vi "Steuerprogramm10-14.vi"() -> ()   [LabVIEW 2010]
uses:
  <vilib>/rvi/interface/nirviReadWriteControl/nirviReadWriteControl.xnode
  <vilib>/rvi/errors/niLvFpgaWhatHappensToTopLevelVI.ctl
  <vilib>/rvi/interface/common/niFpgaNodeNameForErrorReporting.ctl
  <vilib>/rvi/errors/niLvFpgaAdjustHostInterfaceError.vi
  gvbooleschRT.vi
  <vilib>/functionblocks/FB Core/FB Core.xnode
  <vilib>/functionblocks/Counter/Elapsed Timer/Elapsed Timer.vi
  <vilib>/functionblocks/NI_FunctionBlock Libraries.lvlib
  <vilib>/rvi/interface/nirviCloseFPGA/nirviCloseFPGA.xnode
  <vilib>/addons/control/pid/NI_PID_pid.lvlib
  C:/Users/HAGAR-IV/Desktop/Zeugs/Johnny/pertrasgc fpga/FPGA-Programm-10-14.vi
  C:/Users/HAGAR-IV/Desktop/Zeugs/markus/version feb 2012/FPGA Bitfiles/pertrasgcfpga2_FPGATarget_FPGA-Programm-10_16368CB6.lvbitx
  <vilib>/addons/control/pid/pid.llb/PID (DBL Array).vi
  NiFpgaLv.dll
  <vilib>/Utility/error.llb/Error Cluster From Error Code.vi
  <vilib>/FPGAPlugInAG/cRIO-9114/niLvFpga_Close_cRIO-9114.vi
panel:
  in  "Int.Stop2":dbl
  in  "Int.Start2":dbl
  out "Probenvol.2":dbl
  in  "Int.Stop1":dbl
  in  "Int.Start1":dbl
  in  "HorstProbenflußNr.":i32
  out "AIs":dbl[](array[numeric])
  out "Probenvol.1":dbl
  in  "Eingang":T1(array[cluster])=[{"Zykluslängen [s]"=[120.0, 120.0, 120.0, 120.0], "ZeitpktDIOsMod0"=[0.0, 120.0], "ZeitpktDIOsMod1"=[0.0, 60.0, 62.0, 70.0, 120.0], "ZeitpktDIOsMod2A"=[0.0, 120.0], "ZeitpktDIOsMod2B"=[0.0, 60.0, 120.0], "DIOsSPMod0"=[[FALSE], [FALSE]], "DIOsSPMod1"=[[FALSE, FALSE, FALSE, FALSE, FALSE, TRUE, TRUE, FALSE, FALSE, FALSE, TRUE, FALSE, FALSE, FALSE, FALSE, FALSE, FALSE, FALSE], [FALSE, FALSE, FALSE, FALSE, FALSE, FALSE, TRUE, FALSE, FALSE, FALSE, FALSE, FALSE, FALSE, FALSE, FALSE, FALSE, TRUE, FALSE], [FALSE, FALSE, FALSE, FALSE, FALSE, FALSE, TRUE, FALSE, FALSE, FALSE, TRUE, FALSE, FALSE, FALSE, FALSE, FALSE, TRUE, FALSE], [FALSE, FALSE, FALSE, FALSE, FALSE, FALSE, TRUE, FALSE, FALSE, FALSE, TRUE, FALSE, FALSE, FALSE, FALSE, FALSE, FALSE, FALSE], [FALSE, FALSE, FALSE, FALSE, FALSE, FALSE, TRUE, FALSE, FALSE, FALSE, TRUE, FALSE, FALSE, FALSE, FALSE, FALSE, FALSE, FALSE]], "DIOsSPMod2A"=[[FALSE], [FALSE]], "DIOsSPMod2B"=[[FALSE], [FALSE]], "Mod0HorstZeitpkt"=[0.0, 120.0], "Mod1HorstZeitpkt"=[0.0, 59.0, 62.0, 120.0], "Mod2AHorstZeitpkt"=[0.0, 120.0], "Mod2BHorstZeitpkt"=[0.0, 120.0], "HorstSPMod0"=[[0.0], [0.0]], "HorstSPMod1"=[[3.0, 0.0, 0.8], [0.0, 0.0, 0.8], [1.0, 0.0, 0.8], [1.0, 0.0, 0.8]], "HorstSPMod2A"=[[0.0], [0.0]], "HorstSPMod2B"=[[0.0], [0.0]], "LangsameHeizungenSP"=[0.0, 100.0, 100.0, 0.0, 0.0, 0.0], "LHHeizen?"=[FALSE, TRUE, FALSE, FALSE, FALSE, FALSE], "ZPktFPGABoolesch"=[0.0, 62.0, 70.0, 120.0], "FPGABoolesch"=[[FALSE, FALSE, FALSE, FALSE, FALSE, FALSE], [FALSE, FALSE, TRUE, FALSE, FALSE, FALSE], [FALSE, FALSE, FALSE, FALSE, FALSE, FALSE], [FALSE, FALSE, FALSE, FALSE, FALSE, FALSE]], "ZeitpktFPGAPID"=[0.0, 120.0], "FPGAPID"=[[{"proportional gain (Kc)"=1.0, "integral gain (Kc*Ts/Ti)"=1.66796875, "derivative gain (Kc*Td/Ts)"=0.0}, {"proportional gain (Kc)"=1.0, "integral gain (Kc*Ts/Ti)"=1.66796875, "derivative gain (Kc*Td/Ts)"=0.0}, {"proportional gain (Kc)"=5.0, "integral gain (Kc*Ts/Ti)"=0.03515625, "derivative gain (Kc*Td/Ts)"=0.0234375}, {"proportional gain (Kc)"=1.0, "integral gain (Kc*Ts/Ti)"=1.66796875, "derivative gain (Kc*Td/Ts)"=0.0}], [{"proportional gain (Kc)"=1.0, "integral gain (Kc*Ts/Ti)"=1.66796875, "derivative gain (Kc*Td/Ts)"=0.0}, {"proportional gain (Kc)"=1.0, "integral gain (Kc*Ts/Ti)"=1.66796875, "derivative gain (Kc*Td/Ts)"=0.0}, {"proportional gain (Kc)"=5.0, "integral gain (Kc*Ts/Ti)"=0.03515625, "derivative gain (Kc*Td/Ts)"=0.0234375}, {"proportional gain (Kc)"=1.0, "integral gain (Kc*Ts/Ti)"=1.66796875, "derivative gain (Kc*Td/Ts)"=0.0}], [{"proportional gain (Kc)"=0.0, "integral gain (Kc*Ts/Ti)"=0.0, "derivative gain (Kc*Td/Ts)"=0.0}, {"proportional gain (Kc)"=0.0, "integral gain (Kc*Ts/Ti)"=0.0, "derivative gain (Kc*Td/Ts)"=0.0}, {"proportional gain (Kc)"=5.0, "integral gain (Kc*Ts/Ti)"=0.03125, "derivative gain (Kc*Td/Ts)"=0.01953125}, {"proportional gain (Kc)"=0.0, "integral gain (Kc*Ts/Ti)"=0.0, "derivative gain (Kc*Td/Ts)"=0.0}], [{"proportional gain (Kc)"=0.0, "integral gain (Kc*Ts/Ti)"=0.0, "derivative gain (Kc*Td/Ts)"=0.0}, {"proportional gain (Kc)"=0.0, "integral gain (Kc*Ts/Ti)"=0.0, "derivative gain (Kc*Td/Ts)"=0.0}, {"proportional gain (Kc)"=5.0, "integral gain (Kc*Ts/Ti)"=0.03125, "derivative gain (Kc*Td/Ts)"=0.01953125}, {"proportional gain (Kc)"=0.0, "integral gain (Kc*Ts/Ti)"=0.0, "derivative gain (Kc*Td/Ts)"=0.0}], [{"proportional gain (Kc)"=0.0, "integral gain (Kc*Ts/Ti)"=0.0, "derivative gain (Kc*Td/Ts)"=0.0}, {"proportional gain (Kc)"=0.0, "integral gain (Kc*Ts/Ti)"=0.0, "derivative gain (Kc*Td/Ts)"=0.0}, {"proportional gain (Kc)"=5.0, "integral gain (Kc*Ts/Ti)"=0.03125, "derivative gain (Kc*Td/Ts)"=0.01953125}, {"proportional gain (Kc)"=0.0, "integral gain (Kc*Ts/Ti)"=0.0, "derivative gain (Kc*Td/Ts)"=0.0}]], "ZeitpktFPGAFixp"=[0.0, 120.0], "FPGAFixp"=[[3.5, 3.5, 1.800048828125, 0.0, 0.0, 0.0, 2.400146484375, 0.0], [3.5, 3.5, 1.800048828125, 0.0, 0.0, 0.0, 2.400146484375, 0.0]], "ZeitpktMach1"=[0.0, 65.0, 72.0, 110.0, 111.0, 120.0], "TempMach1"=[70.0, 70.0, 150.0, 150.0, 70.0, 70.0], "ZeitpktMach2"=[0.0, 0.0, 120.0], "TempMach2"=[0.0, 0.0, 0.0], "PIDs für \"träge\" Heizungen"=[{"proportional gain (Kc)"=1.0, "integral time (Ti, min)"=0.01, "derivative time (Td, min)"=0.0}, {"proportional gain (Kc)"=5.0, "integral time (Ti, min)"=5.0, "derivative time (Td, min)"=5.0}, {"proportional gain (Kc)"=5.0, "integral time (Ti, min)"=1.0, "derivative time (Td, min)"=5.0}, {"proportional gain (Kc)"=1.0, "integral time (Ti, min)"=0.01, "derivative time (Td, min)"=0.0}, {"proportional gain (Kc)"=1.0, "integral time (Ti, min)"=0.01, "derivative time (Td, min)"=0.0}, {"proportional gain (Kc)"=1.0, "integral time (Ti, min)"=0.01, "derivative time (Td, min)"=0.0}], "Zwangsbedingungen"=[[0.0, 0.0, 0.0, 0.0, 0.0]], "Text0 MS-Datei"="text0", "Info"="info", "wie wird gespeichert?"=0, "Speicherlänge"="100", "Dateien fürs MS schicken?"=FALSE, "Pfad MS-Datei CRIO"=path "c:/"}] {"FPGAPID"."proportional gain (Kc)" format="%.11g"; "FPGAPID"."integral gain (Kc*Ts/Ti)" format="%.11g"; "FPGAPID"."derivative gain (Kc*Td/Ts)" format="%.11g"; "FPGAFixp" format="%.14g"}
  out "Ausgang":T2 {"FPGAPID"."proportional gain (Kc)" format="%.11g"; "FPGAPID"."integral gain (Kc*Ts/Ti)" format="%.11g"; "FPGAPID"."derivative gain (Kc*Td/Ts)" format="%.11g"; "FPGAFixp" format="%.14g"}
  out "Zykluslängen [s]":dbl[](array[numeric])
  in  "Tafel putzen1":bool
  in  "Tafel putzen2":bool
  in  "veränderte Methode benutzen":bool
  out "veränderte Methode":T2 {"FPGAPID"."proportional gain (Kc)" format="%.11g"; "FPGAPID"."integral gain (Kc*Ts/Ti)" format="%.11g"; "FPGAPID"."derivative gain (Kc*Td/Ts)" format="%.11g"; "FPGAFixp" format="%.14g"}
  in  "Methode verändern":bool
  in  "dargestellte Größe 2":i32(ring)=1 items=["T-MainCol3", "T-Trap1", "T-Trap2", "T-Stirling", "T-PreCol1", "T-PreCol2", "T-MainCol1", "T-MainCol2", "T-T-Line2", "T-MI1", "T-MI2", "T-MI3", "T-MI4", "T-MI5", "T-MI6", "F-MFM1", "T-MainCol4", "T-BHorst1", "T-BHorst2", "T-BHorst3", "T-BHorst4", "T-Oven1", "T-Oven2", "T-T-Line1", "F-MFM2", "P-Me-HP", "P-Me-LP", "P-Vac", "Ref-Turbo", "I-MS-AC", "I-Trap1", "I-Trap2", "Mod2/AI0", "Mod2/AI1", "Mod2/AI2", "Mod2/AI3", "Mod2/AI4", "Mod2/AI5", "Mod2/AI6", "Mod2/AI7", "Mod2/AI8", "Mod2/AI9", "Mod2/AI10", "Mod2/AI11", "Mod2/AI12", "Mod2/AI13", "Mod2/AI14", "Mod2/AI15", "Mod2/AI16", "Mod2/AI17", "Mod2/AI18", "Mod2/AI19", "Mod2/AI20", "Mod2/AI21", "Mod2/AI22", "Mod2/AI23", "Mod2/AI24", "Mod2/AI25", "Mod2/AI26", "Mod2/AI27", "Mod2/AI28", "Mod2/AI29", "Mod2/AI30", "Mod2/AI31", "Mod3/AI0", "Mod3/AI1", "Mod3/AI2", "Mod3/AI3", "Mod3/AI4", "Mod3/AI5", "Mod3/AI6", "Mod3/AI7", "Mod3/AI8", "Mod3/AI9", "Mod3/AI10", "Mod3/AI11", "Mod3/AI12", "Mod3/AI13", "Mod3/AI14", "Mod3/AI15", "Mod3/AI16", "Mod3/AI17", "Mod3/AI18", "Mod3/AI19", "Mod3/AI20", "Mod3/AI21", "Mod3/AI22", "Mod3/AI23", "Mod3/AI24", "Mod3/AI25", "Mod3/AI26", "Mod3/AI27", "Mod3/AI28", "Mod3/AI29", "Mod3/AI30", "Mod3/AI31", "U_Widr.Trap1 [V]", "Temp.Trap1 [°C]", "U_Widr.Trap2 [V]", "Temp.Trap2 [°C]", "Temp.Mach1 [°C]", "Temp.Mach2 [°C]", "MFC1B", "PressContr1A", "PressContr1B", "PressContr1C", "MFC1A", "PressContr1D", "MFC1A Integriert"]
  in  "Zeitachse2":i32(ring)=1 items=["Zykluszeit [s] Mod0", "Zykluszeit [s] Mod1", "Zykluszeit [s] Mod2A", "Zykluszeit [s] Mod2B"]
  out "Anzeige2":cluster{dbl[], dbl[]}(graph)
  out "Datum/Zeit":string
  in  "wie wird gespeichert?":u16(ring) items=["Time", "Cycle", "All"]
  in  "Info":string
  in  "Speicherlänge":string
  in  "Dateien fürs MS schicken?":bool
  in  "Pfad MS-Datei CRIO":path
  in  "Text0 MS-Datei":string
  out "ZwangsHorst!":cluster{dbl[]}[](array[cluster])
  out "ZwangsHorst?":cluster{bool[]}[](array[cluster])
  out "ZwangsDIO!":cluster{bool[]}[](array[cluster])
  out "ZwangsDIO?":cluster{bool[]}[](array[cluster])
  out "PIDs für \"träge\" Heizungen":T3(array[cluster])
  out "ZwangsLangsameH!":bool[](array[boolean])
  in  "Heizen?LH":bool[](array[boolean])
  out "Zwangsbedingungen":dbl[][](array[numeric])
  out "Traps/Machs":dbl[](array[numeric])
  out "ZwangsFPGABoolesch!":bool[](array[boolean])
  out "ZwangsFPGABoolesch?":bool[](array[boolean])
  in  "LangsameHeizungenSP":dbl[](array[numeric])
  out "ZwangsLangsameH?":bool[](array[boolean])
  out "Zykluszeiten 0, 1, 2A, 2B":dbl[](array[numeric])
  out "Zyklusnummern 0, 1, 2A, 2B":i32[](array[numeric])
  in  "dargestellte Größe 1":i32(ring)=1 items=["T-MainCol3", "T-Trap1", "T-Trap2", "T-Stirling", "T-PreCol1", "T-PreCol2", "T-MainCol1", "T-MainCol2", "T-T-Line2", "T-MI1", "T-MI2", "T-MI3", "T-MI4", "T-MI5", "T-MI6", "F-MFM1", "T-MainCol4", "T-BHorst1", "T-BHorst2", "T-BHorst3", "T-BHorst4", "T-Oven1", "T-Oven2", "T-T-Line1", "F-MFM2", "P-Me-HP", "P-Me-LP", "P-Vac", "Ref-Turbo", "I-MS-AC", "I-Trap1", "I-Trap2", "Mod2/AI0", "Mod2/AI1", "Mod2/AI2", "Mod2/AI3", "Mod2/AI4", "Mod2/AI5", "Mod2/AI6", "Mod2/AI7", "Mod2/AI8", "Mod2/AI9", "Mod2/AI10", "Mod2/AI11", "Mod2/AI12", "Mod2/AI13", "Mod2/AI14", "Mod2/AI15", "Mod2/AI16", "Mod2/AI17", "Mod2/AI18", "Mod2/AI19", "Mod2/AI20", "Mod2/AI21", "Mod2/AI22", "Mod2/AI23", "Mod2/AI24", "Mod2/AI25", "Mod2/AI26", "Mod2/AI27", "Mod2/AI28", "Mod2/AI29", "Mod2/AI30", "Mod2/AI31", "Mod3/AI0", "Mod3/AI1", "Mod3/AI2", "Mod3/AI3", "Mod3/AI4", "Mod3/AI5", "Mod3/AI6", "Mod3/AI7", "Mod3/AI8", "Mod3/AI9", "Mod3/AI10", "Mod3/AI11", "Mod3/AI12", "Mod3/AI13", "Mod3/AI14", "Mod3/AI15", "Mod3/AI16", "Mod3/AI17", "Mod3/AI18", "Mod3/AI19", "Mod3/AI20", "Mod3/AI21", "Mod3/AI22", "Mod3/AI23", "Mod3/AI24", "Mod3/AI25", "Mod3/AI26", "Mod3/AI27", "Mod3/AI28", "Mod3/AI29", "Mod3/AI30", "Mod3/AI31", "U_Widr.Trap1 [V]", "Temp.Trap1 [°C]", "U_Widr.Trap2 [V]", "Temp.Trap2 [°C]", "Temp.Mach1 [°C]", "Temp.Mach2 [°C]", "MFC1B", "PressContr1A", "PressContr1B", "PressContr1C", "MFC1A", "PressContr1D", "MFC1A Integriert"]
  in  "Zeitachse1":i32(ring)=1 items=["Zykluszeit [s] Mod0", "Zykluszeit [s] Mod1", "Zykluszeit [s] Mod2A", "Zykluszeit [s] Mod2B"]
  out "Anzeige1":cluster{dbl[], dbl[]}(graph)
  out "Big Ben, Methodenzeit, Zykluszeit0, Zykluszeit1, Zykluszeit2A, Zykluszeit2B":dbl[](array[numeric])
  out "MWHorst":dbl[](array[numeric])
  out "HorstSP":dbl[](array[numeric])
  out "Mod1Mod2Mod3/AITrapsMachs1Hz":dbl[](array[numeric])
  in  "global stop RT":bool
  out "Big Ben":dbl
  out "Methodenzeit":dbl
  out "Zyklnum1ges":i32
  out "aktuelle TDMS-Datei":refnum<k34>
  in  "Methodennummer":i32(ring) items=["0"]
  out "Methodenwechsel?":bool
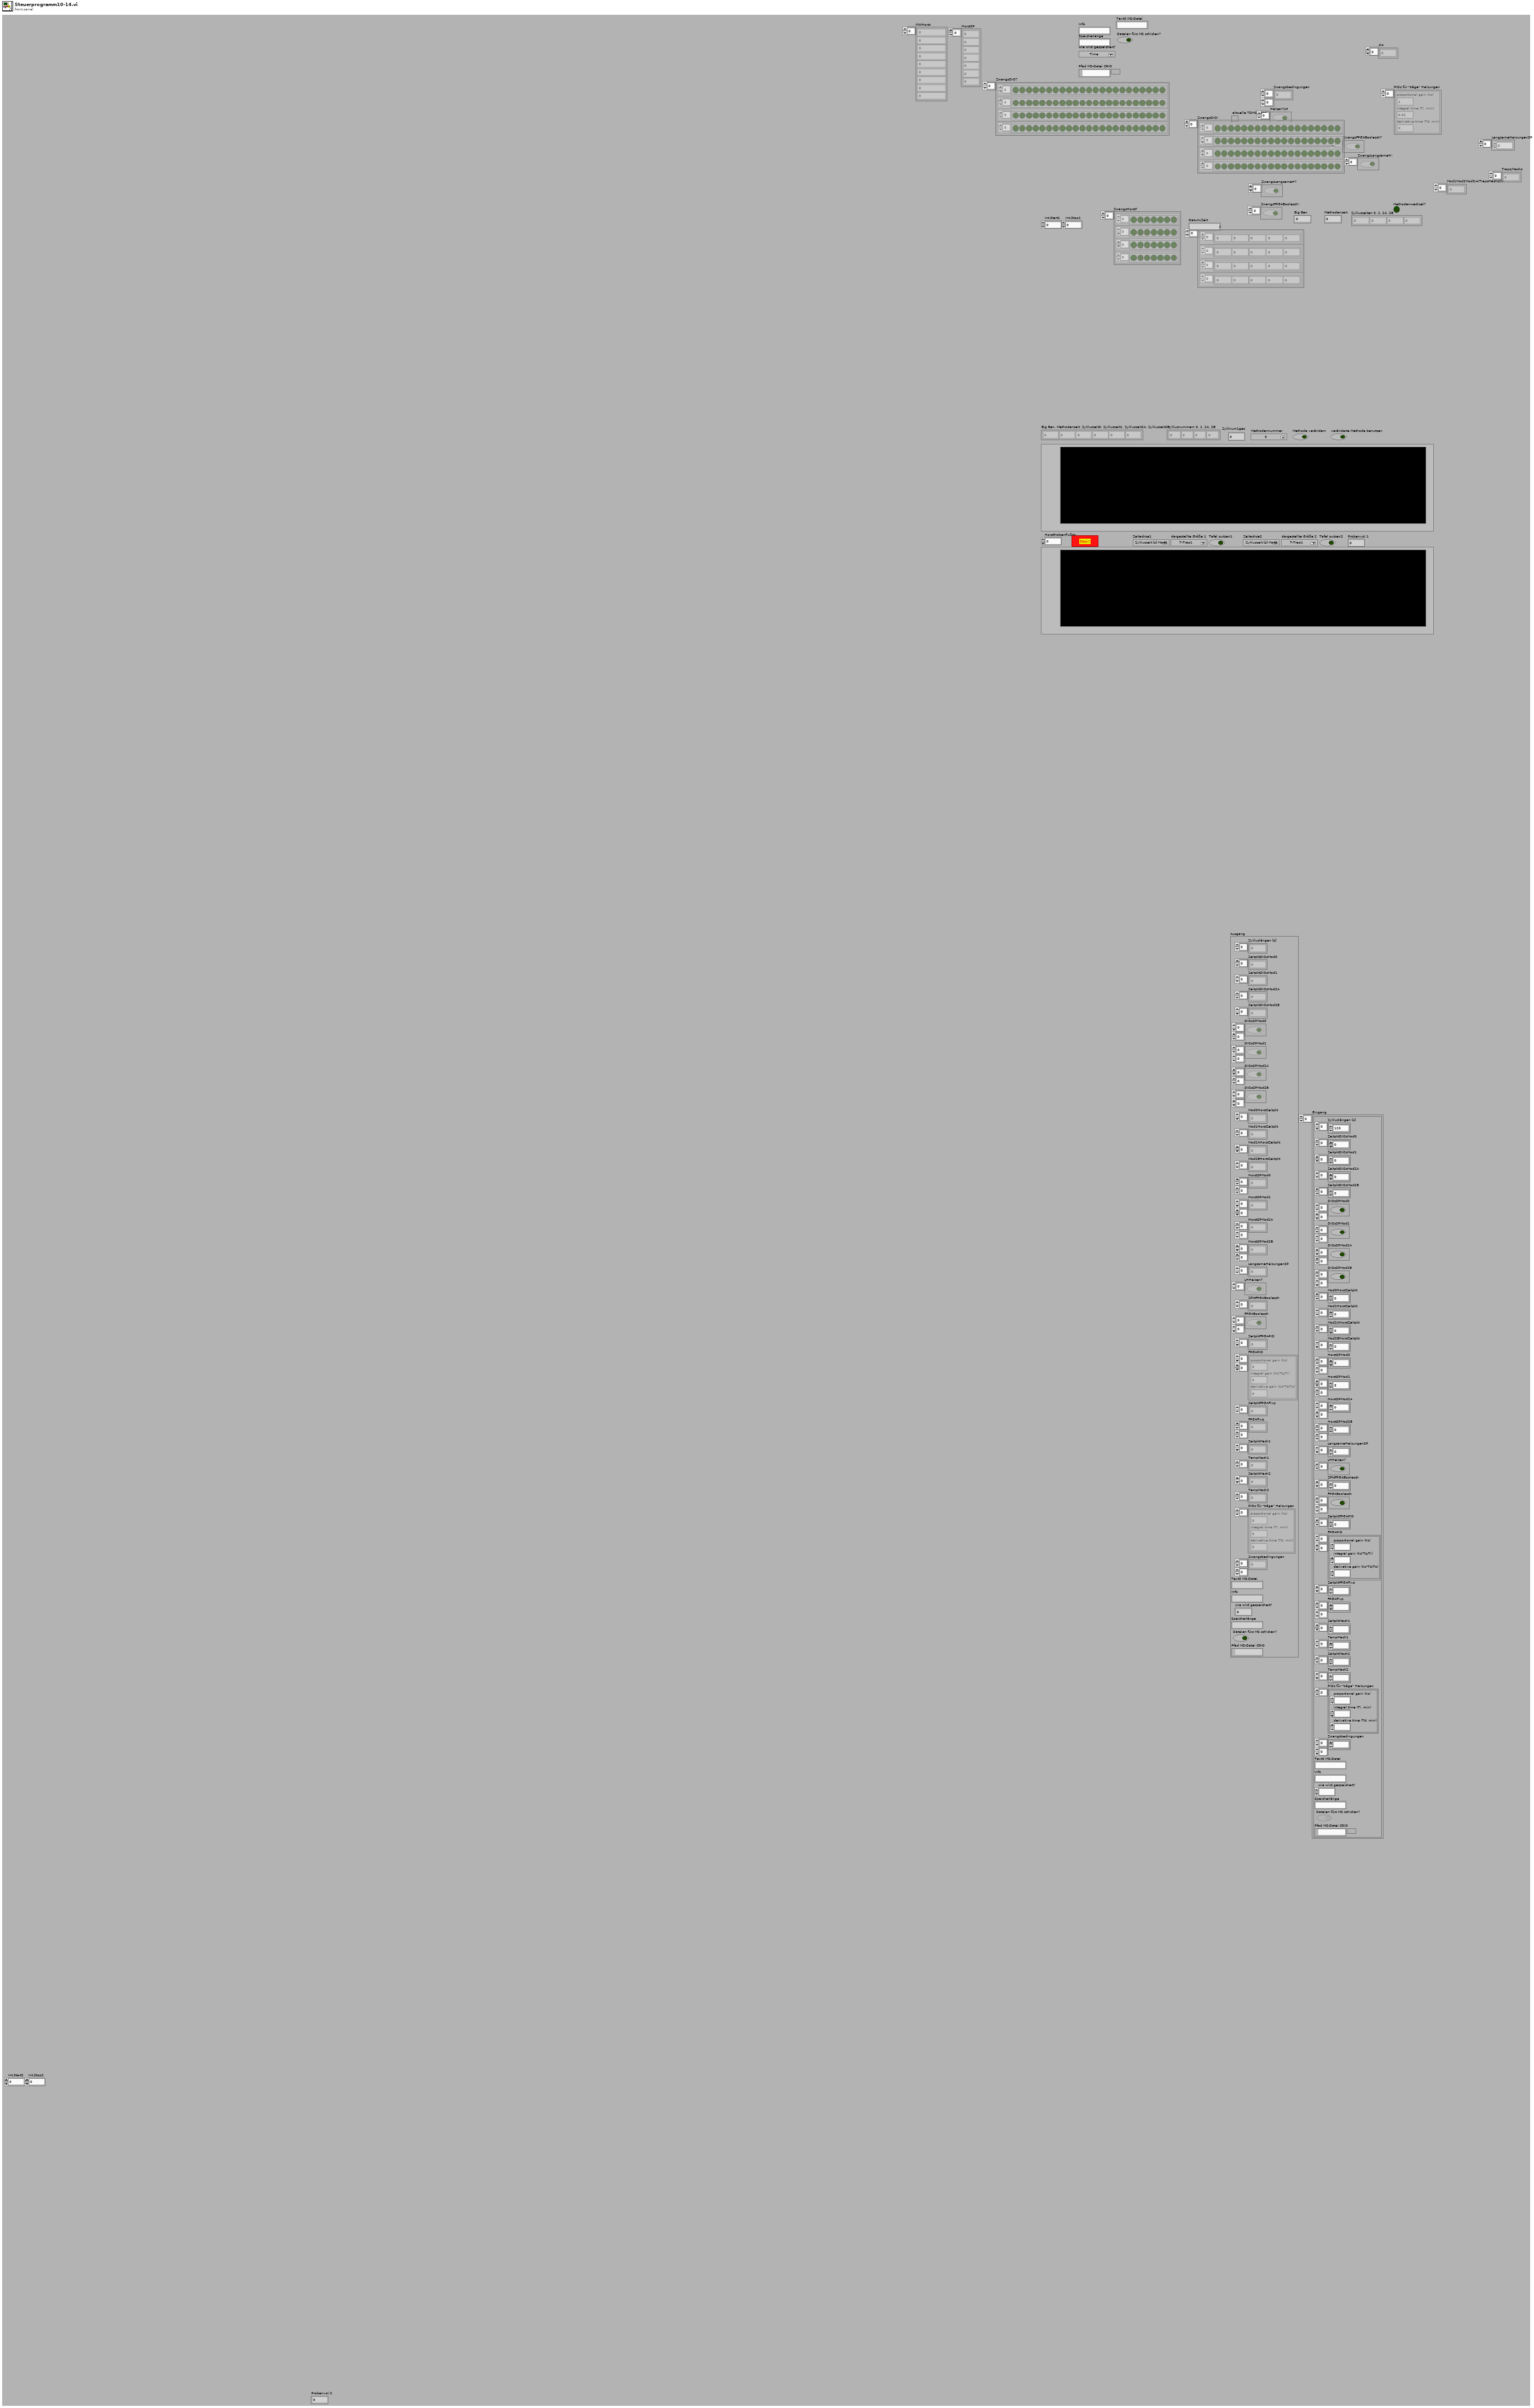
[diagram p1: front panel]
types:
  T1 = cluster{"Zykluslängen [s]":dbl[], "ZeitpktDIOsMod0":dbl[], "ZeitpktDIOsMod1":dbl[], "ZeitpktDIOsMod2A":dbl[], "ZeitpktDIOsMod2B":dbl[], "DIOsSPMod0":bool[][], "DIOsSPMod1":bool[][], "DIOsSPMod2A":bool[][], "DIOsSPMod2B":bool[][], "Mod0HorstZeitpkt":dbl[], "Mod1HorstZeitpkt":dbl[], "Mod2AHorstZeitpkt":dbl[], "Mod2BHorstZeitpkt":dbl[], "HorstSPMod0":dbl[][], "HorstSPMod1":dbl[][], "HorstSPMod2A":dbl[][], "HorstSPMod2B":dbl[][], "LangsameHeizungenSP":dbl[], "LHHeizen?":bool[], "ZPktFPGABoolesch":dbl[], "FPGABoolesch":bool[][], "ZeitpktFPGAPID":dbl[], "FPGAPID":cluster{"proportional gain (Kc)":fxp<+/-,16,8>, "integral gain (Kc*Ts/Ti)":fxp<+/-,16,8>, "derivative gain (Kc*Td/Ts)":fxp<+/-,16,8>}[][], "ZeitpktFPGAFixp":dbl[], "FPGAFixp":fxp<+/-,16,4>[][], "ZeitpktMach1":dbl[], "TempMach1":dbl[], "ZeitpktMach2":dbl[], "TempMach2":dbl[], "PIDs für \"träge\" Heizungen":cluster{"proportional gain (Kc)":dbl, "integral time (Ti, min)":dbl, "derivative time (Td, min)":dbl}[], "Zwangsbedingungen":dbl[][], "Text0 MS-Datei":string, "Info":string, "wie wird gespeichert?":u16, "Speicherlänge":string, "Dateien fürs MS schicken?":bool, "Pfad MS-Datei CRIO":path}[]
  T2 = cluster{"Zykluslängen [s]":dbl[], "ZeitpktDIOsMod0":dbl[], "ZeitpktDIOsMod1":dbl[], "ZeitpktDIOsMod2A":dbl[], "ZeitpktDIOsMod2B":dbl[], "DIOsSPMod0":bool[][], "DIOsSPMod1":bool[][], "DIOsSPMod2A":bool[][], "DIOsSPMod2B":bool[][], "Mod0HorstZeitpkt":dbl[], "Mod1HorstZeitpkt":dbl[], "Mod2AHorstZeitpkt":dbl[], "Mod2BHorstZeitpkt":dbl[], "HorstSPMod0":dbl[][], "HorstSPMod1":dbl[][], "HorstSPMod2A":dbl[][], "HorstSPMod2B":dbl[][], "LangsameHeizungenSP":dbl[], "LHHeizen?":bool[], "ZPktFPGABoolesch":dbl[], "FPGABoolesch":bool[][], "ZeitpktFPGAPID":dbl[], "FPGAPID":cluster{"proportional gain (Kc)":fxp<+/-,16,8>, "integral gain (Kc*Ts/Ti)":fxp<+/-,16,8>, "derivative gain (Kc*Td/Ts)":fxp<+/-,16,8>}[][], "ZeitpktFPGAFixp":dbl[], "FPGAFixp":fxp<+/-,16,4>[][], "ZeitpktMach1":dbl[], "TempMach1":dbl[], "ZeitpktMach2":dbl[], "TempMach2":dbl[], "PIDs für \"träge\" Heizungen":cluster{"proportional gain (Kc)":dbl, "integral time (Ti, min)":dbl, "derivative time (Td, min)":dbl}[], "Zwangsbedingungen":dbl[][], "Text0 MS-Datei":string, "Info":string, "wie wird gespeichert?":u16, "Speicherlänge":string, "Dateien fürs MS schicken?":bool, "Pfad MS-Datei CRIO":path}
  T3 = cluster{"proportional gain (Kc)":dbl, "integral time (Ti, min)":dbl, "derivative time (Td, min)":dbl}[]
  T4 = cluster{"DIOsMod0Nr":i32[], "DIOsMod1Nr":i32[], "DIOsMod2ANr":i32[], "DIOsMod2BNr":i32[], "AIs für \"träge\" Heizungen":i32[], i32[], "AnschlüsseHorstMod0":enum8{"0", "1", "2", "3", "4", "5", "6", "7", "8"}[], "AnschlüsseHorstMod1":enum8{"0", "1", "2", "3", "4", "5", "6", "7", "8"}[], "AnschlüsseHorstMod2A":enum8{"0", "1", "2", "3", "4", "5", "6", "7", "8"}[], "AnschlüsseHorstMod2B":enum8{"0", "1", "2", "3", "4", "5", "6", "7", "8"}[], "StringSPvorgebenMod0":string[], "StringSPvorgebenMod1":string[], "StringSPvorgebenMod2A":string[], "StringSPvorgebenMod2B":string[], "StringMWAntwort0":string[], "StringMWAntwort1":string[], "StringMWAntwort2A":string[], "StringMWAntwort2B":string[], "UmrechnungHorst0":dbl[], "UmrechnungHorst1":dbl[], "UmrechnungHorst2A":dbl[], "UmrechnungHorst2B":dbl[], "StringMWabfragenMod0":string[], "StringMWabfragenMod1":string[], "StringMWabfragenMod2A":string[], "StringMWabfragenMod2B":string[], "Modul1/AI koeff":dbl[][], "Modul2/AI koeff":dbl[][], "Modul3/AI koeff":dbl[][], "Traps/MachKoeff":dbl[][], "AIsNamen":string[], "DIOsMod0Name":string[], "DIOsMod1Name":string[], "DIOsMod2AName":string[], "DIOsMod2BName":string[], "HorstMod0Name":string[], "HorstMod1Name":string[], "HorstMod2AName":string[], "HorstMod2BName":string[], "Startmethode":i32, "Dateiordner Housekeeping":path, "Dateiname Housekeeping":string}
  T5 = enum16{"open", "open or create", "create or replace", "create", "open (read-only)"}
  T6 = enum16{"open", "replace", "create", "open or create", "replace or create", "replace or create with confirmation"}
  T7 = cluster{"Zyklus1":i32, "Zeitachse1":i32, "dargestellte Größe 1":i32, "Zyklus2":i32, "Zeitachse2":i32, "dargestellte Größe 2":i32}
  T8 = typedef "niFpgaNodeNameForErrorReporting.ctl" = enum16{"Open FPGA VI Reference", "Read/Write Control", "Invoke Method: Abort", "Invoke Method: Acknowledge IRQ", "Invoke Method: Download", "Invoke Method: FIFO.Configure", "Invoke Method: FIFO.Read", "Invoke Method: FIFO.Start", "Invoke Method: FIFO.Stop", "Invoke Method: FIFO.Write", "Invoke Method: Reset", "Invoke Method: Run", "Invoke Method: Wait on IRQ", "Close FPGA VI Reference"}
  T9 = typedef "niLvFpgaWhatHappensToTopLevelVI.ctl" = enum16{"top level VI scripted behind XNode", "top level VI inlined behind XNode"}
  T10 = cluster{"DIOsMod0Name":string[], "DIOsMod1Name":string[], "DIOsMod2AName":string[], "DIOsMod2BName":string[], "HorstMod0Name":string[], "HorstMod1Name":string[], "HorstMod2AName":string[], "HorstMod2BName":string[], string[]}
  T11 = cluster{"Zykluslängen [s]":dbl[], "ZeitpktDIOsMod0":dbl[], "ZeitpktDIOsMod1":dbl[], "ZeitpktDIOsMod2A":dbl[], "ZeitpktDIOsMod2B":dbl[], "DIOsSPMod0":bool[][], "DIOsSPMod1":bool[][], "DIOsSPMod2A":bool[][], "DIOsSPMod2B":bool[][], "Mod0HorstZeitpkt":dbl[], "Mod1HorstZeitpkt":dbl[], "Mod2AHorstZeitpkt":dbl[], "Mod2BHorstZeitpkt":dbl[], "HorstSPMod0":dbl[][], "HorstSPMod1":dbl[][], "HorstSPMod2A":dbl[][], "HorstSPMod2B":dbl[][], "LangsameHeizungenSP":dbl[], "LHHeizen?":bool[], "ZPktFPGABoolesch":dbl[], "FPGABoolesch":bool[][], "ZeitpktFPGAPID":dbl[], "FPGAPID":cluster{"proportional gain (Kc)":fxp<+/-,16,8>, "integral gain (Kc*Ts/Ti)":fxp<+/-,16,8>, "derivative gain (Kc*Td/Ts)":fxp<+/-,16,8>}[][], "ZeitpktFPGAFixp":dbl[], "FPGAFixp":fxp<+/-,16,4>[][], "ZeitpktMach1":dbl[], "TempMach1":dbl[], "ZeitpktMach2":dbl[], "TempMach2":dbl[], "PIDs für \"träge\" Heizungen":cluster{"proportional gain (Kc)":dbl, "integral time (Ti, min)":dbl, "derivative time (Td, min)":dbl}[], "Zwangsbedingungen":dbl[][], "Dateien fürs MS schicken?":bool, "ZeitpunkteMPV":dbl[], "SPMPV":i32[], "ZeitpktMSa":dbl, "ZeitpktMSb":dbl, "Int.Start1":dbl, "Int.Stop1":dbl, "Int.Start2":dbl, "Int.Stop2":dbl, "Methodenname":string}
  T12 = cluster{"Heizen?LH[0]":bool, "Heizen?LH[1]":bool, "Heizen?LH[2]":bool, "Heizen?LH[3]":bool, "Heizen?LH[4]":bool, "Heizen?LH[5]":bool}
  T13 = cluster{"[0]":u32, "[1]":u32, "[2]":u32, "[3]":u32, "[4]":u32, "[5]":u32}
  T14 = cluster{"proportional gain (Kc)":fxp<+/-,16,8>, "integral gain (Kc*Ts/Ti)":fxp<+/-,16,8>, "derivative gain (Kc*Td/Ts)":fxp<+/-,16,8>}[][]
  T15 = cluster{cluster{"ZeitpktDIOsMod2B":dbl[]}[], cluster{"DIOsSPMod2B":bool[][]}[], cluster{"Mod2BHorstZeitpkt":dbl[]}[], cluster{"HorstSPMod2B":dbl[][]}[], "LHHeizen?":bool[], "ZPktFPGABoolesch":dbl[], "FPGABoolesch":bool[][], "ZeitpktFPGAPID":dbl[], "FPGAPID":cluster{"proportional gain (Kc)":fxp<+/-,16,8>, "integral gain (Kc*Ts/Ti)":fxp<+/-,16,8>, "derivative gain (Kc*Td/Ts)":fxp<+/-,16,8>}[][], "ZeitpktFPGAFixp":dbl[], "FPGAFixp":fxp<+/-,16,4>[][], "ZeitpktMach1":dbl[], "TempMach1":dbl[], "ZeitpktMach2":dbl[], "TempMach2":dbl[]}
  T16 = cluster{"Zyklusnummern 0, 1, 2A, 2B":i32[], "ZeilennummernDIOs":i32[], "ZwangsDIO?":cluster{bool[]}[], "ZeilennummernHorst":i32[], "ZwangsHorst?":cluster{bool[]}[], "ZeileFPGABoolesch":i32, "ZwangsFPGABoolesch?":bool[], "ZeileFPGAPID":i32, "ZeileFPGAFixp":i32, "ZeileMach1":i32, "ZeileMach2":i32}
  T17 = cluster{"ZyklusnummernSchReg":i32[], "ZeilennummernDIOsSchReg":i32[], "ZwangsDIO?SchReg":cluster{bool[]}[], "ZeilennummernHorstSchReg":i32[], "ZwangsHorst?SchReg":cluster{bool[]}[], "ZeileFPGABooleschSchReg":i32, "ZwangsFPGABoolesch?SchReg":bool[], "ZeileFPGAPIDSchReg":i32, "ZeileFPGAFixpSchReg":i32, "ZeileMach1SchReg":i32, "ZeileMach2SchReg":i32}
  T18 = cluster{string[], string[], string[], dbl[], dbl[], dbl[]}
  T19 = cluster{"Befehle1":string[], "Befehle2":string[], "Befehle3":string[]}
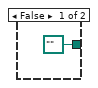
[diagram p2: hidden frame]
diagram:
  (unwired) T1 [{"Zykluslängen [s]"=[180.0, 180.0, 180.0, 180.0], "ZeitpktDIOsMod0"=[0.0, 180.0], "ZeitpktDIOsMod1"=[0.0, 2.0, 15.0, 60.0, 61.0, 70.0, 80.0, 170.0, 180.0], "ZeitpktDIOsMod2A"=[0.0, 180.0], "ZeitpktDIOsMod2B"=[0.0, 60.0, 180.0], "DIOsSPMod0"=[[FALSE], [FALSE]], "DIOsSPMod1"=[[TRUE, TRUE, FALSE, TRUE, FALSE, TRUE, TRUE, TRUE, FALSE, FALSE, TRUE, FALSE, FALSE, FALSE, FALSE, FALSE, FALSE, TRUE], [TRUE, FALSE, FALSE, TRUE, FALSE, TRUE, TRUE, TRUE, FALSE, FALSE, TRUE, FALSE, FALSE, FALSE, FALSE, FALSE, FALSE, TRUE], [TRUE, FALSE, FALSE, FALSE, FALSE, TRUE, TRUE, FALSE, FALSE, FALSE, TRUE, FALSE, FALSE, FALSE, FALSE, FALSE, TRUE, TRUE], [TRUE, FALSE, FALSE, FALSE, FALSE, FALSE, TRUE, FALSE, FALSE, FALSE, TRUE, FALSE, FALSE, FALSE, FALSE, FALSE, TRUE, TRUE], [TRUE, FALSE, FALSE, FALSE, FALSE, FALSE, TRUE, FALSE, FALSE, FALSE, TRUE, FALSE, FALSE, FALSE, FALSE, FALSE, TRUE, TRUE], [TRUE, FALSE, FALSE, FALSE, FALSE, FALSE, TRUE, FALSE, FALSE, FALSE, TRUE, FALSE, FALSE, FALSE, FALSE, FALSE, TRUE, TRUE], [TRUE, FALSE, FALSE, FALSE, FALSE, FALSE, TRUE, FALSE, FALSE, FALSE, TRUE, FALSE, FALSE, FALSE, FALSE, FALSE, FALSE, TRUE], [TRUE, FALSE, FALSE, FALSE, FALSE, FALSE, TRUE, FALSE, FALSE, FALSE, TRUE, FALSE, FALSE, FALSE, FALSE, FALSE, FALSE, TRUE], [TRUE, FALSE, FALSE, FALSE, FALSE, FALSE, TRUE, FALSE, FALSE, FALSE, TRUE, FALSE, FALSE, FALSE, FALSE, FALSE, FALSE, TRUE]], "DIOsSPMod2A"=[[FALSE], [FALSE]], "DIOsSPMod2B"=[[FALSE], [FALSE]], "Mod0HorstZeitpkt"=[0.0, 180.0], "Mod1HorstZeitpkt"=[0.0, 55.0, 75.0, 180.0], "Mod2AHorstZeitpkt"=[0.0, 20.0, 180.0], "Mod2BHorstZeitpkt"=[0.0, 380.0], "HorstSPMod0"=[[2.66], [2.66]], "HorstSPMod1"=[[1.9, 0.0, 1.2], [0.0, 0.0, 1.2], [1.9, 0.0, 1.2], [1.9, 0.0, 1.2]], "HorstSPMod2A"=[[300.0], [300.0], [300.0]], "HorstSPMod2B"=[[0.0], [0.0]], "LangsameHeizungenSP"=[60.0, 220.0, 120.0, 60.0, 110.0, 0.0], "LHHeizen?"=[FALSE, TRUE, TRUE, FALSE, TRUE, FALSE], "ZPktFPGABoolesch"=[0.0, 60.0, 75.0, 180.0], "FPGABoolesch"=[[FALSE, FALSE, FALSE, FALSE, TRUE, FALSE], [FALSE, FALSE, TRUE, FALSE, TRUE, FALSE], [FALSE, FALSE, FALSE, FALSE, TRUE, FALSE], [FALSE, FALSE, FALSE, FALSE, TRUE, FALSE]], "ZeitpktFPGAPID"=[0.0, 60.0, 180.0], "FPGAPID"=[[{"proportional gain (Kc)"=5.0, "integral gain (Kc*Ts/Ti)"=0.0, "derivative gain (Kc*Td/Ts)"=0.0}, {"proportional gain (Kc)"=1.0, "integral gain (Kc*Ts/Ti)"=1.66796875, "derivative gain (Kc*Td/Ts)"=0.0}, {"proportional gain (Kc)"=5.0, "integral gain (Kc*Ts/Ti)"=0.03515625, "derivative gain (Kc*Td/Ts)"=0.0234375}, {"proportional gain (Kc)"=1.0, "integral gain (Kc*Ts/Ti)"=1.66796875, "derivative gain (Kc*Td/Ts)"=0.0}], [{"proportional gain (Kc)"=5.0, "integral gain (Kc*Ts/Ti)"=0.0, "derivative gain (Kc*Td/Ts)"=0.0}, {"proportional gain (Kc)"=1.0, "integral gain (Kc*Ts/Ti)"=1.66796875, "derivative gain (Kc*Td/Ts)"=0.0}, {"proportional gain (Kc)"=5.0, "integral gain (Kc*Ts/Ti)"=0.03515625, "derivative gain (Kc*Td/Ts)"=0.0234375}, {"proportional gain (Kc)"=1.0, "integral gain (Kc*Ts/Ti)"=1.66796875, "derivative gain (Kc*Td/Ts)"=0.0}], [{"proportional gain (Kc)"=0.0, "integral gain (Kc*Ts/Ti)"=0.0, "derivative gain (Kc*Td/Ts)"=0.0}, {"proportional gain (Kc)"=0.0, "integral gain (Kc*Ts/Ti)"=0.0, "derivative gain (Kc*Td/Ts)"=0.0}, {"proportional gain (Kc)"=2.0, "integral gain (Kc*Ts/Ti)"=0.03125, "derivative gain (Kc*Td/Ts)"=0.01953125}, {"proportional gain (Kc)"=0.0, "integral gain (Kc*Ts/Ti)"=0.0, "derivative gain (Kc*Td/Ts)"=0.0}], [{"proportional gain (Kc)"=0.0, "integral gain (Kc*Ts/Ti)"=0.0, "derivative gain (Kc*Td/Ts)"=0.0}, {"proportional gain (Kc)"=0.0, "integral gain (Kc*Ts/Ti)"=0.0, "derivative gain (Kc*Td/Ts)"=0.0}, {"proportional gain (Kc)"=2.0, "integral gain (Kc*Ts/Ti)"=0.03125, "derivative gain (Kc*Td/Ts)"=0.01953125}, {"proportional gain (Kc)"=0.0, "integral gain (Kc*Ts/Ti)"=0.0, "derivative gain (Kc*Td/Ts)"=0.0}], [{"proportional gain (Kc)"=0.0, "integral gain (Kc*Ts/Ti)"=0.0, "derivative gain (Kc*Td/Ts)"=0.0}, {"proportional gain (Kc)"=0.0, "integral gain (Kc*Ts/Ti)"=0.0, "derivative gain (Kc*Td/Ts)"=0.0}, {"proportional gain (Kc)"=2.0, "integral gain (Kc*Ts/Ti)"=0.03125, "derivative gain (Kc*Td/Ts)"=0.01953125}, {"proportional gain (Kc)"=0.0, "integral gain (Kc*Ts/Ti)"=0.0, "derivative gain (Kc*Td/Ts)"=0.0}]], "ZeitpktFPGAFixp"=[0.0, 60.0, 75.0, 180.0], "FPGAFixp"=[[0.0, 0.0, 0.0, 0.0, 0.0, 0.0, 2.85009765625, 0.0], [4.59423828125, 4.599365234375, 1.699951171875, 0.0, 0.0, 0.0, 2.85009765625, 0.0], [0.0, 0.0, 0.0, 0.0, 0.0, 0.0, 2.85009765625, 0.0], [0.0, 0.0, 0.0, 0.0, 0.0, 0.0, 2.85009765625, 0.0]], "ZeitpktMach1"=[0.0, 1.0, 100.0, 101.0, 177.0, 178.0, 180.0], "TempMach1"=[50.0, 50.0, 50.0, 250.0, 250.0, 50.0, 50.0], "ZeitpktMach2"=[0.0, 0.0, 120.0], "TempMach2"=[0.0, 0.0, 0.0], "PIDs für \"träge\" Heizungen"=[{"proportional gain (Kc)"=1.0, "integral time (Ti, min)"=0.01, "derivative time (Td, min)"=0.0}, {"proportional gain (Kc)"=2.0, "integral time (Ti, min)"=1.0, "derivative time (Td, min)"=0.0}, {"proportional gain (Kc)"=4.0, "integral time (Ti, min)"=1.0, "derivative time (Td, min)"=0.0}, {"proportional gain (Kc)"=1.0, "integral time (Ti, min)"=0.01, "derivative time (Td, min)"=0.0}, {"proportional gain (Kc)"=2.0, "integral time (Ti, min)"=0.0, "derivative time (Td, min)"=0.0}, {"proportional gain (Kc)"=1.0, "integral time (Ti, min)"=0.01, "derivative time (Td, min)"=0.0}], "Zwangsbedingungen"=[[3.0, 4.0, 100.0, 23.0, 4.0, 200.0, 0.0, 0.0]], "Text0 MS-Datei"="text0", "Info"="info", "wie wird gespeichert?"=0, "Speicherlänge"="100", "Dateien fürs MS schicken?"=FALSE, "Pfad MS-Datei CRIO"=path "c:/"}] ("Eingang 2")
  (unwired) T4 {"DIOsMod0Nr"=[32], "DIOsMod1Nr"=[5, 6, 7, 10, 11, 14, 15, 16, 17, 18, 20, 23, 25, 26, 27, 28, 29, 30], "DIOsMod2ANr"=[33], "DIOsMod2BNr"=[34], "AIs für \"träge\" Heizungen"=[17, 6, 0, 19, 21, 23], [1, 3, 1, 1], "AnschlüsseHorstMod0"=[enum."1"], "AnschlüsseHorstMod1"=[enum."1", enum."1", enum."1"], "AnschlüsseHorstMod2A"=[enum."1"], "AnschlüsseHorstMod2B"=[enum."1"], "StringSPvorgebenMod0"=[":060A020121"], "StringSPvorgebenMod1"=[":060B020121", ":0618020121", ":060D020121"], "StringSPvorgebenMod2A"=[":0619020121"], "StringSPvorgebenMod2B"=[":060C020121"], "StringMWAntwort0"=[":060A020121"], "StringMWAntwort1"=[":060B020121", ":0618020121", ":060D020121"], "StringMWAntwort2A"=[":0619020121"], "StringMWAntwort2B"=[":060C020121"], "UmrechnungHorst0"=[0.0003125], "UmrechnungHorst1"=[9.375e-05, 9.375e-05, 9.375e-05], "UmrechnungHorst2A"=[0.046875], "UmrechnungHorst2B"=[9.375e-05], "StringMWabfragenMod0"=[":060A0401210120"], "StringMWabfragenMod1"=[":060B0401210120", ":06180401210120", ":060D0401210120"], "StringMWabfragenMod2A"=[":06190401210120"], "StringMWabfragenMod2B"=[":060C0401210120"], "Modul1/AI koeff"=[[-249.333, 111.873, 2.1471], [-249.333, 111.873, 2.1471], [-249.333, 111.873, 2.1471], [-249.333, 111.873, 2.1471], [-237.2852, -153.162, 6.0782], [-237.2852, -153.162, 6.0782], [-249.333, 111.873, 2.1471], [-249.333, 111.873, 2.1471], [-249.333, 111.873, 2.1471], [-249.333, 111.873, 2.1471], [-249.333, 111.873, 2.1471], [-249.333, 111.873, 2.1471], [-249.333, 111.873, 2.1471], [-249.333, 111.873, 2.1471], [-249.333, 111.873, 2.1471], [0.0, 1.0, 0.0], [-249.333, 111.873, 2.1471], [-249.333, 111.873, 2.1471], [-249.333, 111.873, 2.1471], [-249.333, 111.873, 2.1471], [-249.333, 111.873, 2.1471], [-249.333, 111.873, 2.1471], [-249.333, 111.873, 2.1471], [-249.333, 111.873, 2.1471], [0.0, 1.0, 0.0], [0.0, 1.0, 0.0], [0.0, 1.0, 0.0], [0.0, 1.0, 0.0], [0.0, 1.0, 0.0], [0.0, 1.0, 0.0], [0.0, 1.0, 0.0], [0.0, 1.0, 0.0]], "Modul2/AI koeff"=[[0.0, 1.0, 0.0], [0.0, 1.0, 0.0], [0.0, 1.0, 0.0], [0.0, 1.0, 0.0], [0.0, 1.0, 0.0], [0.0, 1.0, 0.0], [0.0, 1.0, 0.0], [0.0, 1.0, 0.0], [0.0, 1.0, 0.0], [0.0, 1.0, 0.0], [0.0, 1.0, 0.0], [0.0, 1.0, 0.0], [0.0, 1.0, 0.0], [0.0, 1.0, 0.0], [0.0, 1.0, 0.0], [0.0, 1.0, 0.0], [0.0, 1.0, 0.0], [0.0, 1.0, 0.0], [0.0, 1.0, 0.0], [0.0, 1.0, 0.0], [0.0, 1.0, 0.0], [0.0, 1.0, 0.0], [0.0, 1.0, 0.0], [0.0, 1.0, 0.0], [0.0, 1.0, 0.0], [0.0, 1.0, 0.0], [0.0, 1.0, 0.0], [0.0, 1.0, 0.0], [0.0, 1.0, 0.0], [0.0, 1.0, 0.0], [0.0, 1.0, 0.0], [0.0, 1.0, 0.0]], "Modul3/AI koeff"=[[0.0, 1.0, 0.0], [0.0, 1.0, 0.0], [0.0, 1.0, 0.0], [0.0, 1.0, 0.0], [0.0, 1.0, 0.0], [0.0, 1.0, 0.0], [0.0, 1.0, 0.0], [0.0, 1.0, 0.0], [0.0, 1.0, 0.0], [0.0, 1.0, 0.0], [0.0, 1.0, 0.0], [0.0, 1.0, 0.0], [0.0, 1.0, 0.0], [0.0, 1.0, 0.0], [0.0, 1.0, 0.0], [0.0, 1.0, 0.0], [0.0, 1.0, 0.0], [0.0, 1.0, 0.0], [0.0, 1.0, 0.0], [0.0, 1.0, 0.0], [0.0, 1.0, 0.0], [0.0, 1.0, 0.0], [0.0, 1.0, 0.0], [0.0, 1.0, 0.0], [0.0, 1.0, 0.0], [0.0, 1.0, 0.0], [0.0, 1.0, 0.0], [0.0, 1.0, 0.0], [0.0, 1.0, 0.0], [0.0, 1.0, 0.0], [0.0, 1.0, 0.0], [0.0, 1.0, 0.0]], "Traps/MachKoeff"=[[0.0, 1.0, 0.0], [-249.333, 111.873, 2.1471], [0.0, 1.0, 0.0], [-249.333, 111.873, 2.1471], [-237.2852, 153.1621, 6.0782], [-237.2852, 153.1621, 6.0782]], "AIsNamen"=["T-MainCol3", "T-Trap1", "T-Trap2", "T-Stirling", "T-PreCol1", "T-PreCol2", "T-MainCol1", "T-MainCol2", "T-T-Line2", "T-MI1", "T-MI2", "T-MI3", "T-MI4", "T-MI5", "T-MI6", "F-MFM1", "T-MainCol4", "T-BHorst1", "T-BHorst2", "T-BHorst3", "T-BHorst4", "T-Oven1", "T-Oven2", "T-T-Line1", "F-MFM2", "P-Me-HP", "P-Me-LP", "P-Vac", "Ref-Turbo", "I-MS-AC", "I-Trap1", "I-Trap2", "Mod2/AI0", "Mod2/AI1", "Mod2/AI2", "Mod2/AI3", "Mod2/AI4", "Mod2/AI5", "Mod2/AI6", "Mod2/AI7", "Mod2/AI8", "Mod2/AI9", "Mod2/AI10", "Mod2/AI11", "Mod2/AI12", "Mod2/AI13", "Mod2/AI14", "Mod2/AI15", "Mod2/AI16", "Mod2/AI17", "Mod2/AI18", "Mod2/AI19", "Mod2/AI20", "Mod2/AI21", "Mod2/AI22", "Mod2/AI23", "Mod2/AI24", "Mod2/AI25", "Mod2/AI26", "Mod2/AI27", "Mod2/AI28", "Mod2/AI29", "Mod2/AI30", "Mod2/AI31", "Mod3/AI0", "Mod3/AI1", "Mod3/AI2", "Mod3/AI3", "Mod3/AI4", "Mod3/AI5", "Mod3/AI6", "Mod3/AI7", "Mod3/AI8", "Mod3/AI9", "Mod3/AI10", "Mod3/AI11", "Mod3/AI12", "Mod3/AI13", "Mod3/AI14", "Mod3/AI15", "Mod3/AI16", "Mod3/AI17", "Mod3/AI18", "Mod3/AI19", "Mod3/AI20", "Mod3/AI21", "Mod3/AI22", "Mod3/AI23", "Mod3/AI24", "Mod3/AI25", "Mod3/AI26", "Mod3/AI27", "Mod3/AI28", "Mod3/AI29", "Mod3/AI30", "Mod3/AI31"], "DIOsMod0Name"=["blindDIO0"], "DIOsMod1Name"=["on/off P-MS", "MS Start", "MS Stop", "FanMach1", "FanReserve", "Valve1A", "on/off PrePump", "S1Reserve", "on/off VacP2", "on/off VacP1", "S1D", "FanMach2", "S1C", "on/off Stirling", "S1B", "S1A", "Valve1B", "on/off Turbo"], "DIOsMod2AName"=["blindDIO2A"], "DIOsMod2BName"=["blindDIO2B"], "HorstMod0Name"=["MFC1B"], "HorstMod1Name"=["PressContr1A", "PressContr1B", "PressContr1C"], "HorstMod2AName"=["MFC1A"], "HorstMod2BName"=["PressContr1D"], "Startmethode"=0, "Dateiordner Housekeeping"=path "C:/", "Dateiname Housekeeping"="test"} ("Einstellungen")
  n1 = flat-sequence {
    tunnel: [w40] -> w31
    tunnel: [w65] -> w30
    tunnel: [w109] -> w29
    tunnel: [w110] -> w28
    tunnel: [w108] -> w24
    tunnel: [w85] -> w23
    tunnel: [w99] -> w22
    tunnel: [w74] -> w21
    tunnel: [w90] -> w20
    tunnel: [w105] -> w19
    tunnel: [w69] -> w18
    tunnel: [w68] -> w17
    tunnel: [w48] -> w16
    tunnel: [w107] -> w15
    tunnel: [w104] -> w14
    tunnel: T4 {"DIOsMod0Nr"=[32], "DIOsMod1Nr"=[5, 6, 7, 10, 11, 14, 15, 16, 17, 18, 20, 23, 25, 26, 27, 28, 29, 30], "DIOsMod2ANr"=[33], "DIOsMod2BNr"=[34], "AIs für \"träge\" Heizungen"=[17, 6, 0, 19, 21, 23], [1, 3, 1, 1], "AnschlüsseHorstMod0"=[enum."1"], "AnschlüsseHorstMod1"=[enum."1", enum."1", enum."1"], "AnschlüsseHorstMod2A"=[enum."1"], "AnschlüsseHorstMod2B"=[enum."1"], "StringSPvorgebenMod0"=[":060A020121"], "StringSPvorgebenMod1"=[":060B020121", ":0618020121", ":060D020121"], "StringSPvorgebenMod2A"=[":0519010104"], "StringSPvorgebenMod2B"=[":060C020121 "], "StringMWAntwort0"=[":060A020121"], "StringMWAntwort1"=[":060B020121", ":0618020121", ":060D020121"], "StringMWAntwort2A"=[":0619020121"], "StringMWAntwort2B"=[":060C020121"], "UmrechnungHorst0"=[0.0003125], "UmrechnungHorst1"=[9.375e-05, 9.375e-05, 9.375e-05], "UmrechnungHorst2A"=[1.0], "UmrechnungHorst2B"=[9.375e-05], "StringMWabfragenMod0"=[":060A0401210120"], "StringMWabfragenMod1"=[":060B0401210120", ":06180401210120", ":060D0401210120"], "StringMWabfragenMod2A"=[":06190401210120"], "StringMWabfragenMod2B"=[":060C0401210120"], "Modul1/AI koeff"=[[-249.333, 111.873, 2.1471], [-249.333, 111.873, 2.1471], [-249.333, 111.873, 2.1471], [-249.333, 111.873, 2.1471], [-237.2852, -153.162, 6.0782], [-237.2852, -153.162, 6.0782], [-249.333, 111.873, 2.1471], [-249.333, 111.873, 2.1471], [-249.333, 111.873, 2.1471], [-249.333, 111.873, 2.1471], [-249.333, 111.873, 2.1471], [-249.333, 111.873, 2.1471], [-249.333, 111.873, 2.1471], [-249.333, 111.873, 2.1471], [-249.333, 111.873, 2.1471], [0.0, 1.0, 0.0], [-249.333, 111.873, 2.1471], [-249.333, 111.873, 2.1471], [-249.333, 111.873, 2.1471], [-249.333, 111.873, 2.1471], [-249.333, 111.873, 2.1471], [-249.333, 111.873, 2.1471], [-249.333, 111.873, 2.1471], [-249.333, 111.873, 2.1471], [0.0, 1.0, 0.0], [0.0, 1.0, 0.0], [0.0, 1.0, 0.0], [0.0, 1.0, 0.0], [0.0, 1.0, 0.0], [0.0, 1.0, 0.0], [0.0, 1.0, 0.0], [0.0, 1.0, 0.0]], "Modul2/AI koeff"=[[0.0, 1.0, 0.0], [0.0, 1.0, 0.0], [0.0, 1.0, 0.0], [0.0, 1.0, 0.0], [0.0, 1.0, 0.0], [0.0, 1.0, 0.0], [0.0, 1.0, 0.0], [0.0, 1.0, 0.0], [0.0, 1.0, 0.0], [0.0, 1.0, 0.0], [0.0, 1.0, 0.0], [0.0, 1.0, 0.0], [0.0, 1.0, 0.0], [0.0, 1.0, 0.0], [0.0, 1.0, 0.0], [0.0, 1.0, 0.0], [0.0, 1.0, 0.0], [0.0, 1.0, 0.0], [0.0, 1.0, 0.0], [0.0, 1.0, 0.0], [0.0, 1.0, 0.0], [0.0, 1.0, 0.0], [0.0, 1.0, 0.0], [0.0, 1.0, 0.0], [0.0, 1.0, 0.0], [0.0, 1.0, 0.0], [0.0, 1.0, 0.0], [0.0, 1.0, 0.0], [0.0, 1.0, 0.0], [0.0, 1.0, 0.0], [0.0, 1.0, 0.0], [0.0, 1.0, 0.0]], "Modul3/AI koeff"=[[0.0, 1.0, 0.0], [0.0, 1.0, 0.0], [0.0, 1.0, 0.0], [0.0, 1.0, 0.0], [0.0, 1.0, 0.0], [0.0, 1.0, 0.0], [0.0, 1.0, 0.0], [0.0, 1.0, 0.0], [0.0, 1.0, 0.0], [0.0, 1.0, 0.0], [0.0, 1.0, 0.0], [0.0, 1.0, 0.0], [0.0, 1.0, 0.0], [0.0, 1.0, 0.0], [0.0, 1.0, 0.0], [0.0, 1.0, 0.0], [0.0, 1.0, 0.0], [0.0, 1.0, 0.0], [0.0, 1.0, 0.0], [0.0, 1.0, 0.0], [0.0, 1.0, 0.0], [0.0, 1.0, 0.0], [0.0, 1.0, 0.0], [0.0, 1.0, 0.0], [0.0, 1.0, 0.0], [0.0, 1.0, 0.0], [0.0, 1.0, 0.0], [0.0, 1.0, 0.0], [0.0, 1.0, 0.0], [0.0, 1.0, 0.0], [0.0, 1.0, 0.0], [0.0, 1.0, 0.0]], "Traps/MachKoeff"=[[0.0, 1.0, 0.0], [-249.333, 111.873, 2.1471], [0.0, 1.0, 0.0], [-249.333, 111.873, 2.1471], [-237.2852, 153.1621, 6.0782], [-237.2852, 153.1621, 6.0782]], "AIsNamen"=["T-MainCol3", "T-Trap1", "T-Trap2", "T-Stirling", "T-PreCol1", "T-PreCol2", "T-MainCol1", "T-MainCol2", "T-T-Line2", "T-MI1", "T-MI2", "T-MI3", "T-MI4", "T-MI5", "T-MI6", "F-MFM1", "T-MainCol4", "T-BHorst1", "T-BHorst2", "T-BHorst3", "T-BHorst4", "T-Oven1", "T-Oven2", "T-T-Line1", "F-MFM2", "P-Me-HP", "P-Me-LP", "P-Vac", "Ref-Turbo", "I-MS-AC", "I-Trap1", "I-Trap2", "Mod2/AI0", "Mod2/AI1", "Mod2/AI2", "Mod2/AI3", "Mod2/AI4", "Mod2/AI5", "Mod2/AI6", "Mod2/AI7", "Mod2/AI8", "Mod2/AI9", "Mod2/AI10", "Mod2/AI11", "Mod2/AI12", "Mod2/AI13", "Mod2/AI14", "Mod2/AI15", "Mod2/AI16", "Mod2/AI17", "Mod2/AI18", "Mod2/AI19", "Mod2/AI20", "Mod2/AI21", "Mod2/AI22", "Mod2/AI23", "Mod2/AI24", "Mod2/AI25", "Mod2/AI26", "Mod2/AI27", "Mod2/AI28", "Mod2/AI29", "Mod2/AI30", "Mod2/AI31", "Mod3/AI0", "Mod3/AI1", "Mod3/AI2", "Mod3/AI3", "Mod3/AI4", "Mod3/AI5", "Mod3/AI6", "Mod3/AI7", "Mod3/AI8", "Mod3/AI9", "Mod3/AI10", "Mod3/AI11", "Mod3/AI12", "Mod3/AI13", "Mod3/AI14", "Mod3/AI15", "Mod3/AI16", "Mod3/AI17", "Mod3/AI18", "Mod3/AI19", "Mod3/AI20", "Mod3/AI21", "Mod3/AI22", "Mod3/AI23", "Mod3/AI24", "Mod3/AI25", "Mod3/AI26", "Mod3/AI27", "Mod3/AI28", "Mod3/AI29", "Mod3/AI30", "Mod3/AI31"], "DIOsMod0Name"=["blindDIO0"], "DIOsMod1Name"=["on/off P-MS", "MS Start", "MS Stop", "FanMach1", "FanReserve", "Valve1A", "on/off PrePump", "Air-In", "on/off VacP2", "on/off VacP1", "S1D", "FanMach2", "S1C", "on/off Stirling", "S1B", "S1A", "Valve1B", "on/off Turbo"], "DIOsMod2AName"=["blindDIO2A"], "DIOsMod2BName"=["blindDIO2B"], "HorstMod0Name"=["MFC1B"], "HorstMod1Name"=["PressContr1A", "PressContr1B", "PressContr1C"], "HorstMod2AName"=["MFC1A"], "HorstMod2BName"=["PressContr1D"], "Startmethode"=0, "Dateiordner Housekeeping"=path "C:/data", "Dateiname Housekeeping"="test"} ("Einstellungen") -> [w106]
    tunnel: [w84] -> w13
    tunnel: "Eingang" -> [w77]
    tunnel: [w66] -> w12
    tunnel: [w64] -> w11
    tunnel: [w63] -> w10
    tunnel: [w53] -> w9
    tunnel: [w43] -> w6
    tunnel: [w42] -> w5
    tunnel: [w41] -> w4
    tunnel: [w36] -> w3
    tunnel: [w35] -> w2
    tunnel: [w34] -> w1
    tunnel: w31 -> [w149]
    tunnel: w30 -> [w222]
    tunnel: w29 -> [w221]
    tunnel: w28 -> [w220]
    tunnel: [w218] -> w27
    tunnel: [w217] -> w26
    tunnel: [w149] -> w25
    tunnel: w24 -> [_]
    tunnel: w23 -> [w157]
    tunnel: w22 -> [w156]
    tunnel: w21 -> [w158]
    tunnel: w20 -> [w155]
    tunnel: w19 -> [w151]
    tunnel: w18 -> [w214]
    tunnel: w17 -> [w211]
    tunnel: w16 -> [w213]
    tunnel: w15 -> [w212]
    tunnel: w14 -> [w169]
    tunnel: "Eingang" -> [w205]
    tunnel: w13 -> [w203]
    tunnel: w12 -> [w208]
    tunnel: w11 -> [w207]
    tunnel: w10 -> [w206]
    tunnel: w9 -> [w204]
    tunnel: w6 -> [w201]
    tunnel: w5 -> [w200]
    tunnel: w4 -> [w199]
    tunnel: w3 -> [w198]
    tunnel: w2 -> [w197]
    tunnel: w1 -> [w196]
    tunnel: w27 -> [w693]
    tunnel: w26 -> [w692]
    tunnel: w25 -> [w691]
    frame #0 {
      w79 = string[] ["U_Widr.Trap1 [V]", "Temp.Trap1 [°C]", "U_Widr.Trap2 [V]", "Temp.Trap2 [°C]", "Temp.Mach1 [°C]", "Temp.Mach2 [°C]"]
      w82 = string[] ["Big Ben [s]", "Methodenzeit [s]", "Zykluszeit [s] Mod0", "Zykluszeit [s] Mod1", "Zykluszeit [s] Mod2A", "Zykluszeit [s] Mod2B"]
      w107 = 6  # AnzahlLH
      w49 = FALSE ("Undefinierte Werte möglich")
      w51 = FALSE ("global stop RT")
      w113 = "z"
      w115 = "m"
      w116 = ".tdms" ("String")
      n2 = global write "gvbooleschRT.vi" "global stop RT"(w51) -> ()
      n3 = property on="dargestellte Größe 2" class="Ring (strict)"("AllowUndefVals"=w49) -> ()  [unwired: 2 in, 2 out]
      n4 = property on="Zeitachse2" class="Ring (strict)"("AllowUndefVals"=w49) -> ()  [unwired: 2 in, 2 out]
      n5 = property on="Zeitachse1" class="Ring (strict)"("AllowUndefVals"=w49) -> ()  [unwired: 2 in, 2 out]
      n6 = property on="dargestellte Größe 1" class="Ring (strict)"("AllowUndefVals"=w49) -> ()  [unwired: 2 in, 2 out]
      n7 = property on="Methodennummer" class="Ring (strict)"("AllowUndefVals"=w49) -> ()  [unwired: 2 in, 2 out]
      n8 = Array Size(array=w77) -> (size(s)=w76:i32)
      n9 = for {
        N: w76 -> [_]
        tunnel: [w138] -> w75 mode=indexing
        i -> [w139]
        n10 = Number To Decimal String(number=w139) -> (decimal integer string=w138:string)  [unwired: 1 in]
      }
      n11 = case shown="True" "Dateien fürs MS schicken?" {
        tunnel: [path "" ("path") w126] -> w66
        frame False {
        }
        frame True {
          n12 = Open/Create/Replace File(file path (use dialog)="Pfad MS-Datei CRIO", operation (0:open)=T6."replace or create" ("Operation (0:Öffnen)")) -> (refnum out=w135:refnum<file>, error out=w134:errorcluster)  [unwired: 4 in, 1 out]
          n13 = Open/Create/Replace File(file path (use dialog)=path "c:/fromcriordy.txt" ("Dateipfad (Dialog verwenden)"), operation (0:open)=T6."replace or create" ("Operation (0:Öffnen)")) -> (refnum out=w129:refnum<file>, error out=w130:errorcluster)  [unwired: 4 in, 1 out]
          n14 = Write to Text File(file (use dialog)=w135, text="Text0 MS-Datei", error in=w134) -> (refnum out=w132:refnum<file>, error out=w131:errorcluster)  [unwired: 1 in, 1 out]
          n15 = Close File(refnum=w129, error in=w130) -> (path=w126:path)  [unwired: 1 out]
          n16 = Close File(refnum=w132, error in=w131) -> ()  [unwired: 2 out]
        }
      }
      n17 = local write "global stop RT"(w51) -> ()
      n18 = call "FPGA-Start.vi"() -> ("error out"=w108:errorcluster, "FPGA VI Reference Out"=w40:refnum<k20>)  [unwired: 2 in]
      n19 = Number To Decimal String(number=0 ("Wert")) -> (decimal integer string=w117:string)  [unwired: 1 in]
      n20 = Number To Decimal String(number=1 ("Wert")) -> (decimal integer string=w112:string)  [unwired: 1 in]
      n21 = property on="Methodennummer" class="Ring (strict)"("Strings []"=w75) -> ()  [unwired: 2 in, 2 out]
      n22 = Unbundle(w106) -> ("DIOsMod0Nr"=w73:i32[], "DIOsMod1Nr"=w72:i32[], "DIOsMod2ANr"=w71:i32[], "DIOsMod2BNr"=w70:i32[], "AIs für \"träge\" Heizungen"=w105:i32[], w104:i32[], "StringSPvorgebenMod0"=w103:string[], "StringSPvorgebenMod1"=w102:string[], "StringSPvorgebenMod2A"=w101:string[], "StringSPvorgebenMod2B"=w100:string[], "StringMWAntwort0"=w98:string[], "StringMWAntwort1"=w97:string[], "StringMWAntwort2A"=w96:string[], "StringMWAntwort2B"=w95:string[], "UmrechnungHorst0"=w94:dbl[], "UmrechnungHorst1"=w93:dbl[], "UmrechnungHorst2A"=w92:dbl[], "UmrechnungHorst2B"=w91:dbl[], "StringMWabfragenMod0"=w89:string[], "StringMWabfragenMod1"=w88:string[], "StringMWabfragenMod2A"=w87:string[], "StringMWabfragenMod2B"=w86:string[], "Modul1/AI koeff"=w39:dbl[][], "Modul2/AI koeff"=w38:dbl[][], "Modul3/AI koeff"=w37:dbl[][], "Traps/MachKoeff"=w44:dbl[][], "AIsNamen"=w80:string[], "DIOsMod0Name"=w62:string[], "DIOsMod1Name"=w61:string[], "DIOsMod2AName"=w60:string[], "DIOsMod2BName"=w59:string[], "HorstMod0Name"=w58:string[], "HorstMod1Name"=w57:string[], "HorstMod2AName"=w56:string[], "HorstMod2BName"=w55:string[], "Startmethode"=w65:i32, "Dateiordner Housekeeping"=w63:path, "Dateiname Housekeeping"=w64:string)  [unwired: 4 out]
      n23 = Number To Decimal String(number=w65) -> (decimal integer string=w114:string)  [unwired: 1 in]
      n24 = property on="Methodennummer" class="Ring (strict)"("Value"=w65) -> ()  [unwired: 2 in, 2 out]
      n25 = Concatenate Strings(w64, w115, w114, w113, w117, w116) -> (w121:string)
      n26 = Concatenate Strings(w64, w115, w114, w113, w112, w116) -> (w120:string)
      n27 = Build Path(base path=w63, name or relative path=w121) -> (appended path=w122:path)
      n28 = Build Path(base path=w63, name or relative path=w120) -> (appended path=w111:path)
      n29 = Build Array (concatenate)(w58, w57, w56, w55) -> (w78:string[])
      n30 = Build Array (concatenate)(w103, w102, w101, w100) -> (w99:string[])
      n31 = TDMS Open(10:T5."create" ("Operation (0:Öffnen)"), 11:w122) -> (3:w109:refnum<k34>)  [unwired: 4 in, 1 out]
      n32 = Build Array (concatenate)(w89, w88, w87, w86) -> (w85:string[])
      n33 = Build Array (concatenate)(w98, w97, w96, w95) -> (w90:string[])
      n34 = local write "aktuelle TDMS-Datei"(w109) -> ()
      n35 = Add Array Elements(numeric array=w104) -> (sum=w48:i32)
      n36 = Build Array (concatenate)(w94, w93, w92, w91) -> (w74:dbl[])
      n37 = Split 1D Array(array=w82, index=2 ("Index")) -> (second subarray=w52:string[])  [unwired: 1 out]
      n38 = property on="Zeitachse1" class="Ring (strict)"("Strings []"=w52) -> ()  [unwired: 2 in, 2 out]
      n39 = property on="Zeitachse2" class="Ring (strict)"("Strings []"=w52) -> ()  [unwired: 2 in, 2 out]
      n40 = Build Array (concatenate)(w80, w79, w78) -> (w50:string[])
      n41 = Index Array(array=w44, index (col)=2 ("Deaktivierter Index (Spalte)")) -> (element=w43:dbl[])  [unwired: 1 in]
      n42 = Index Array(array=w44, index (col)=1 ("Deaktivierter Index (Spalte)")) -> (element=w42:dbl[])  [unwired: 1 in]
      n43 = Index Array(array=w44, index (col)=0 ("Deaktivierter Index (Spalte)")) -> (element=w41:dbl[])  [unwired: 1 in]
      n44 = call "AIKoeffSortieren.vi"("Modul3/AI koeff"=w37, "Modul2/AI koeff"=w38, "Modul1/AI koeff"=w39) -> ("P0"=w34:dbl[], "P1"=w35:dbl[], "P2"=w36:dbl[])
      n45 = Build Cluster Array(w73, w72, w71, w70) -> (w69:cluster{"DIOsMod2BNr":i32[]}[])
      n46 = for {
        tunnel: w69 -> [w141] mode=indexing
        tunnel: [w142] -> w68 mode=indexing
        n47 = Unbundle(w141) -> ("DIOsMod2BNr"=w140:i32[])
        n48 = Array Size(array=w140) -> (size(s)=w142:i32)
      }
      n49 = property on="dargestellte Größe 1" class="Ring (strict)"("Strings []"=w50) -> ()  [unwired: 2 in, 2 out]
      n50 = property on="dargestellte Größe 2" class="Ring (strict)"("Strings []"=w50) -> ()  [unwired: 2 in, 2 out]
      n51 = Bundle("DIOsMod0Name"=w62, "DIOsMod1Name"=w61, "DIOsMod2AName"=w60, "DIOsMod2BName"=w59, "HorstMod0Name"=w58, "HorstMod1Name"=w57, "HorstMod2AName"=w56, "HorstMod2BName"=w55, string[] ["Horst1", "MainCol1", "MainCol2", "Horst2", "Oven", "T-Line"]) -> (w53:T10)  [unwired: 1 in]
      n52 = TDMS Open(10:T5."create" ("Operation (0:Öffnen)"), 11:w111) -> (3:w110:refnum<k34>)  [unwired: 4 in, 1 out]
      n53 = Build Array (concatenate)(string[] ["Datei Nr.", "Zyklusnr. Mod0", "Zyklusnr. Mod1", "Zyklusnr. Mod2A", "Zyklusnr. Mod2B"], w82, w80, w79, w78, "Probenvolumen1", "Probenvolumen2") -> (w84:string[])
    }
    frame #1 {
      w143 = FALSE
      w144 = 0.0
      w147 = dbl[] []
      w175 = 0
      w173 = string[] []
      n54 = while {
        shift-right: ["Methodennummer"] -> _
        shift-left: w222 -> [w684]
        stop <- w686 stop-if-true
        n55 = call "Warten"("Count(mSec)"=u32 1000) -> ()  [unwired: 1 out]
        n56 = Not Equal?(x=w684, y="Methodennummer") -> (x != y?=→"Methodenwechsel?":bool)
        n57 = global read "gvbooleschRT.vi" "global stop RT"() -> (w686:bool)
      }
      n58 = while {
        tunnel: w205 -> [w417]
        tunnel: w204 -> [w414]
        stop <- w418 stop-if-true
        n59 = local read "Methodennummer"() -> (w416:i32)
        n60 = Index Array(array=w417, index=w416) -> (element=w415:T2)
        n61 = while {
          shift-right: [w420] -> _
          shift-left: w415 -> [w421]
          tunnel: w414 -> [w419]
          stop <- w424 stop-if-true
          n62 = local read "Methodenwechsel?"() -> (w426:bool)
          n63 = global read "gvbooleschRT.vi" "global stop RT"() -> (w425:bool)
          n64 = call "Warten19"("Count(mSec)"=u32 500) -> ()  [unwired: 1 out]
          n65 = case shown="True" "Methode verändern" {
            tunnel: w421 -> [w427 w431]
            tunnel: [w427 w430] -> w420
            tunnel: w419 -> [_ w428]
            frame False {
            }
            frame True {
              n66 = call "methodeändern.vi"("Methode"=w431, "Namen"=w428) -> ("Methode"=w430:T11)  [unwired: 1 in]
              "Ausgang" <- w430
              n67 = property on="Methode verändern" class="Bool (strict)"("Value"=FALSE ("Methode verändern")) -> ()  [unwired: 2 in, 2 out]
            }
          }
          "veränderte Methode" <- w420
          n68 = Or(x=w426, y=w425) -> (x .or. y?=w424:bool)
        }
        n69 = global read "gvbooleschRT.vi" "global stop RT"() -> (w418:bool)
      }
      n70 = Add Array Elements(numeric array=w211) -> (sum=w210:i32)
      n71 = while {
        stop <- w462 stop-if-true
        w453 = 10.0
        n72 = local read "Traps/Machs"() -> (w455:dbl[])
        n73 = call "Warten27"("Count(mSec)"=u32 1000) -> ()  [unwired: 1 out]
        n74 = local read "AIs"() -> (w460:dbl[])
        n75 = for {
          N: 9 -> [_]
          shift-right: [w465] -> w458
          shift-left: w460 -> [w466]
          shift-right: [w463] -> w454
          shift-left: w455 -> [w464]
          n76 = flat-sequence {
            tunnel: w466 -> [w473]
            tunnel: [w471] -> w465
            tunnel: w464 -> [w469]
            tunnel: [w468] -> w463
            frame #0 {
              n77 = call "Warten28"("Count(mSec)"=u32 100) -> ()  [unwired: 1 out]
            }
            frame #1 {
              n78 = local read "AIs"() -> (w472:dbl[])
              n79 = local read "Traps/Machs"() -> (w470:dbl[])
              n80 = Add(x=w473, y=w472) -> (x+y=w471:dbl[])
              n81 = Add(x=w470, y=w469) -> (x+y=w468:dbl[])
            }
          }
        }
        n82 = Divide(x=w458, y=w453) -> (x/y=w457:dbl[])
        n83 = Divide(x=w454, y=w453) -> (x/y=w452:dbl[])
        n84 = Build Array (concatenate)(w457, w452) -> (→"Mod1Mod2Mod3/AITrapsMachs1Hz":dbl[])
        n85 = global read "gvbooleschRT.vi" "global stop RT"() -> (w462:bool)
      }
      n86 = Array Size(array=w151) -> (size(s)=w148:i32)
      n87 = while {
        tunnel: w149 -> [w367]
        tunnel: w198 -> [w365]
        tunnel: w197 -> [w364]
        tunnel: w196 -> [w363]
        stop <- w368 stop-if-true
        n88 = call "AIsFIFORT.vi"("P0"=w363, "P1"=w364, "P2"=w365, "FPGA VI Reference In"=w367) -> (0:→"AIs")
        n89 = global read "gvbooleschRT.vi" "global stop RT"() -> (w368:bool)
      }
      n90 = Initialize Array(cluster{"output high":dbl, "output low":dbl} {"output high"=99999.0, "output low"=0.0} ("output range"), w148) -> (w150:cluster{"output high":dbl, "output low":dbl}[])
      n91 = while {
        tunnel: w151 -> [w260]
        tunnel: w150 -> [w262]
        tunnel: w149 -> [w257]
        stop <- w265 stop-if-true
        n92 = local read "AIs"() -> (w261:dbl[])
        n93 = call "Warten4"("Count(mSec)"=u32 100) -> ()  [unwired: 1 out]
        n94 = for {
          tunnel: w261 -> [w339]
          tunnel: w260 -> [w338] mode=indexing
          tunnel: [w337] -> w259 mode=indexing
          n95 = Index Array(array=w339, index=w338) -> (element=w337:dbl)
        }
        n96 = local read "PIDs für \"träge\" Heizungen"() -> (w263:T3)
        n97 = call-poly <vilib>:"PID.vi"("output range"=w262, "PID gains"=w263, "process variable"=w259, "setpoint"="LangsameHeizungenSP") -> ("output"=w258:dbl[])  [unwired: 6 in, 1 out]
        n98 = To Unsigned Long Integer(number=w258) -> (unsigned 32bit integer=w255:u32[])
        n99 = Array To Cluster(array="Heizen?LH") -> (cluster=w256:T12)
        n100 = Array To Cluster(array=w255) -> (cluster=w254:T13)
        n101 = xnode "Read/Write Control"("FPGA VI Reference In"=w257, "LHHeizen?"=w256, "LHPulse(us)"=w254) -> ()  [unwired: 1 in, 2 out]
        n102 = global read "gvbooleschRT.vi" "global stop RT"() -> (w265:bool)
      }
      n103 = while {
        tunnel: w211 -> [w485]
        tunnel: w213 -> [w486]
        tunnel: w212 -> [w487]
        tunnel: w169 -> [w484]
        tunnel: w210 -> [w493]
        stop <- "global stop RT" stop-if-true
        n104 = local read "Mod1Mod2Mod3/AITrapsMachs1Hz"() -> (w490:dbl[])
        n105 = call "Warten5"("Count(mSec)"=u32 1000) -> ()  [unwired: 1 out]
        n106 = local read "Zwangsbedingungen"() -> (w488:dbl[][])
        n107 = local read "Methodennummer"() -> (w491:i32)
        n108 = local read "MWHorst"() -> (w489:dbl[])
        n109 = call "Zwangsbedingungen.vi"("AnzahlDIOs"=w493, "global stop RT"="global stop RT", "Methodennummer"=w491, "Mod1Mod2Mod3/AITrapsMachs1Hz"=w490, "MWHorst"=w489, "Zwangsbedingungen"=w488, "AnzahlLH"=w487, "AnzahlHorst"=w486, "AnzahlDIOs/Modul"=w485, "AnzahlHorst/Modul"=w484) -> ("ZwangsFPGABoolesch?"=→"ZwangsFPGABoolesch?":bool[], "ZwangsFPGABoolesch!"=→"ZwangsFPGABoolesch!":bool[], "Methodennummer"=w481:i32, "global stop RT"=w480:bool, "ZwangsDIO?"=→"ZwangsDIO?":cluster{bool[]}[], "ZwangsDIO!"=→"ZwangsDIO!":cluster{bool[]}[], "ZwangsLangsameH?"=→"ZwangsLangsameH?":bool[], "ZwangsLangsameH!"=→"ZwangsLangsameH!":bool[], "ZwangsHorst?"=→"ZwangsHorst?":cluster{bool[]}[], "ZwangsHorst!"=→"ZwangsHorst!":cluster{dbl[]}[])
        n110 = global write "gvbooleschRT.vi" "global stop RT"("global stop RT") -> ()
        n111 = local write "global stop RT"(w480) -> ()
        n112 = local write "Methodennummer"(w481) -> ()
      }
      n113 = Bundle(w147, w147, w147, w147) -> (w146:cluster{dbl[], dbl[], dbl[], dbl[]})  [unwired: 1 in]
      n114 = while {
        shift-right: [w226] -> _
        shift-left: w146 -> [w228]
        shift-right: [w225] -> _
        shift-left: w146 -> [w227]
        shift-right: [w223] -> _
        shift-left: T7 {"Zyklus1"=0, "Zeitachse1"=0, "dargestellte Größe 1"=0, "Zyklus2"=0, "Zeitachse2"=0, "dargestellte Größe 2"=0} ("AnzeigeEinstellungen") -> [w224]
        stop <- w251 stop-if-true
        w232 = 0.0 ("X-Achse.Bereich:Minimum")
        n115 = call "Warten6"("Count(mSec)"=u32 100) -> ()  [unwired: 1 out]
        n116 = local read "Big Ben, Methodenzeit, Zykluszeit0, Zykluszeit1, Zykluszeit2A, Zykluszeit2B"() -> (w231:dbl[])
        n117 = property on="Anzeige1" class="XYGraph (strict)"("XScale.Minimum"=w232) -> ()  [unwired: 2 in, 2 out]
        n118 = property on="Anzeige2" class="XYGraph (strict)"("XScale.Minimum"=w232) -> ()  [unwired: 2 in, 2 out]
        n119 = local read "veränderte Methode benutzen"() -> (w242:bool)
        n120 = local read "Zyklusnummern 0, 1, 2A, 2B"() -> (w230:i32[])
        n121 = local read "Methodenwechsel?"() -> (w241:bool)
        n122 = local read "Zykluslängen [s]"() -> (w234:dbl[])
        n123 = local read "Traps/Machs"() -> (w237:dbl[])
        n124 = local read "MWHorst"() -> (w236:dbl[])
        n125 = local read "AIs"() -> (w238:dbl[])
        n126 = call "Anzeige.vi"("AIs"=w238, "Zykluslängen [s]"=w234, "Cluster1"=w228, "veränderte Methode benutzen"=w242, "Big Ben, Methodenzeit, Zykluszeit0, Zykluszeit1, Zykluszeit2A, Zykluszeit2B"=w231, "Zyklusnummern 0, 1, 2A, 2B"=w230, "Cluster2"=w227, "AnzeigeEinstellungen"=w224, "Tafel putzen2"="Tafel putzen2", "Tafel putzen1"="Tafel putzen1", "MWHorst"=w236, "Traps/Machs"=w237, "dargestellte Größe 1"="dargestellte Größe 1", "Zeitachse1"="Zeitachse1", "Zeitachse2"="Zeitachse2", "dargestellte Größe 2"="dargestellte Größe 2", "Methodenwechsel?"=w241) -> ("Anzeige2"=→"Anzeige2":cluster{dbl[], dbl[]}, "Cluster1"=w226:cluster{dbl[], dbl[], dbl[], dbl[]}, "x1Inkr"=w248:dbl, "Cluster2"=w225:cluster{dbl[], dbl[], dbl[], dbl[]}, "Anzeige1"=→"Anzeige1":cluster{dbl[], dbl[]}, "AnzeigeEinstellungen"=w223:T7, "x2Max"=w233:dbl, "x2Inkr"=w235:dbl, "x1Max"=w249:dbl)  [unwired: 2 in]
        n127 = global read "gvbooleschRT.vi" "global stop RT"() -> (w251:bool)
        n128 = property on="Anzeige1" class="XYGraph (strict)"("XScale.Increment"=w248) -> ()  [unwired: 2 in, 2 out]
        n129 = property on="Anzeige2" class="XYGraph (strict)"("XScale.Maximum"=w233) -> ()  [unwired: 2 in, 2 out]
        n130 = property on="Anzeige2" class="XYGraph (strict)"("XScale.Increment"=w235) -> ()  [unwired: 2 in, 2 out]
        n131 = property on="Anzeige1" class="XYGraph (strict)"("XScale.Maximum"=w249) -> ()  [unwired: 2 in, 2 out]
      }
      n132 = while {
        stop <- w433 stop-if-true
        n133 = call "Warten17"("Count(mSec)"=u32 1000 ("Zu wartende ms")) -> ()  [unwired: 1 out]
        n134 = Get Date/Time In Seconds() -> (seconds since 1Jan1904=w435:timestamp)
        n135 = Format Date/Time String(time format string (%c)="%Y%m%d%H%M%S" ("Zeitformatierungs-String (%c)"), seconds (now)=w435) -> (date/time string=→"Datum/Zeit":string)  [unwired: 1 in]
        n136 = global read "gvbooleschRT.vi" "global stop RT"() -> (w433:bool)
      }
      n137 = while {
        tunnel: w149 -> [w369]
        tunnel: w201 -> [w374]
        tunnel: w200 -> [w371]
        tunnel: w199 -> [w370]
        stop <- w375 stop-if-true
        n138 = call "TrapsMachMitteln.vi"("Traps/MachKoeff0"=w370, "Traps/MachKoeff1"=w371, "Traps/MachKoeff2"=w374, "FPGA VI Reference In"=w369) -> (0:→"Traps/Machs")
        n139 = global read "gvbooleschRT.vi" "global stop RT"() -> (w375:bool)
        n140 = call "Warten25"("Count(mSec)"=u32 100) -> ()  [unwired: 1 out]
      }
      n141 = while "Methoden- und Zyklussteuerung" {
        shift-right: [w570] -> _
        shift-left: 0.0 -> [w569]
        shift-right: [w568] -> _
        shift-left: -1 -> [w567]
        tunnel: w149 -> [w563]
        tunnel: w214 -> [w564]
        tunnel: w205 -> [w562]
        i -> [w573]
        stop <- w574 stop-if-true
        w509 = 0  # ZeileMach2
        w510 = 0  # ZeileMach1
        w511 = 0  # ZeileFPGAFixp
        w512 = 0  # ZeileFPGAPID
        w514 = 0  # ZeileFPGABoolesch
        w516 = i32[] [0, 0, 0, 0]  # ZeilennummernHorst
        w518 = i32[] [0, 0, 0, 0]  # ZeilennummernDIOs
        n142 = local read "Methodennummer"() -> (w561:i32)
        n143 = Add(x=w567, y=1) -> (x+y=w565:i32)
        n144 = Index Array(array=w562, index=w561) -> (element=w538:T2)
        n145 = local read "veränderte Methode benutzen"() -> (w536:bool)
        n146 = case shown="True" w536 {
          tunnel: w538 -> [w575 _]
          tunnel: [w575 w577] -> w537
          frame False {
          }
          frame True {
            n147 = property on="veränderte Methode benutzen" class="Bool (strict)"("Value"=FALSE ("Methode verändern")) -> ()  [unwired: 2 in, 2 out]
            n148 = local read "veränderte Methode"() -> (w577:T2)
          }
        }
        n149 = Unbundle(w537) -> ("Zykluslängen [s]"=w560:dbl[], "ZeitpktDIOsMod0"=w548:dbl[], "ZeitpktDIOsMod1"=w547:dbl[], "ZeitpktDIOsMod2A"=w546:dbl[], "ZeitpktDIOsMod2B"=w545:dbl[], "DIOsSPMod0"=w552:bool[][], "DIOsSPMod1"=w551:bool[][], "DIOsSPMod2A"=w550:bool[][], "DIOsSPMod2B"=w549:bool[][], "Mod0HorstZeitpkt"=w556:dbl[], "Mod1HorstZeitpkt"=w555:dbl[], "Mod2AHorstZeitpkt"=w554:dbl[], "Mod2BHorstZeitpkt"=w553:dbl[], "HorstSPMod0"=w507:dbl[][], "HorstSPMod1"=w502:dbl[][], "HorstSPMod2A"=w501:dbl[][], "HorstSPMod2B"=w500:dbl[][], "LangsameHeizungenSP"=w559:dbl[], "LHHeizen?"=w531:bool[], "ZPktFPGABoolesch"=w530:dbl[], "FPGABoolesch"=w529:bool[][], "ZeitpktFPGAPID"=w528:dbl[], "FPGAPID"=w527:T14, "ZeitpktFPGAFixp"=w526:dbl[], "FPGAFixp"=w525:fxp<+/-,16,4>[][], "ZeitpktMach1"=w524:dbl[], "TempMach1"=w523:dbl[], "ZeitpktMach2"=w522:dbl[], "TempMach2"=w521:dbl[], "PIDs für \"träge\" Heizungen"=→"PIDs für \"träge\" Heizungen":T3, "Zwangsbedingungen"=→"Zwangsbedingungen":dbl[][], "Text0 MS-Datei"=w544:string, "Info"=w543:string, "wie wird gespeichert?"=w542:u16, "Speicherlänge"=w541:string, "Dateien fürs MS schicken?"=w540:bool, "Pfad MS-Datei CRIO"=w539:path)
        "Zykluslängen [s]" <- w560
        n150 = local write "LangsameHeizungenSP"(w559) -> ()
        n151 = local write "Text0 MS-Datei"(w544) -> ()
        n152 = local write "Info"(w543) -> ()
        n153 = local write "wie wird gespeichert?"(w542) -> ()
        n154 = local write "Speicherlänge"(w541) -> ()
        n155 = local write "Dateien fürs MS schicken?"(w540) -> ()
        n156 = local write "Pfad MS-Datei CRIO"(w539) -> ()
        n157 = Equal?(x=w573, y=0) -> (x = y?=w571:bool)
        n158 = local read "Zyklusnummern 0, 1, 2A, 2B"() -> (w519:i32[])
        n159 = while "Zeit" {
          tunnel: w571 -> [w619]
          tunnel: [w613] -> w570
          tunnel: w569 -> [w618]
          tunnel: [w606] -> w568
          tunnel: w565 -> [w607]
          tunnel: w560 -> [w615]
          i -> [w622]
          stop <- w602 stop-if-true
          n160 = Equal?(x=w622, y=0) -> (x = y?=w620:bool)
          n161 = call "Warten3"("Count(mSec)"=u32 50) -> ()  [unwired: 1 out]
          n162 = And(x=w619, y=w620) -> (x .and. y?=w624:bool)
          n163 = xnode "Elapsed Timer"("reset"=w624) -> ("elapsed time (ms)"=w627:i32)  [unwired: 2 in, 1 out]
          n164 = local read "veränderte Methode benutzen"() -> (w604:bool)
          n165 = local read "Methodenwechsel?"() -> (w617:bool)
          n166 = global read "gvbooleschRT.vi" "global stop RT"() -> (w616:bool)
          n167 = To Double Precision Float(number=w627) -> (double precision float=w626:dbl)
          n168 = Or(x=w617, y=w616) -> (x .or. y?=w603:bool)
          n169 = Divide(x=w626, y=1000.0) -> (x/y=w613:dbl)
          "Big Ben" <- w613
          n170 = Or(x=w604, y=w603) -> (x .or. y?=w602:bool)
          n171 = Subtract(x=w613, y=w618) -> (x-y=w612:dbl)
          "Methodenzeit" <- w612
          n172 = for {
            tunnel: w615 -> [w630] mode=indexing
            tunnel: w612 -> [w631]
            tunnel: [w629] -> w614 mode=indexing
            tunnel: [w628] -> w611 mode=indexing
            n173 = Quotient & Remainder(x=w631, y=w630) -> (x-y*floor(x/y)=w629:dbl, floor(x/y)=w628:dbl)
          }
          "Zykluszeiten 0, 1, 2A, 2B" <- w614
          n174 = Build Array (concatenate)(w613, w612, w614) -> (w605:dbl[])
          n175 = To Long Integer(number=w611) -> (32bit integer=w610:i32[])
          "Zyklusnummern 0, 1, 2A, 2B" <- w610
          n176 = local write "Big Ben, Methodenzeit, Zykluszeit0, Zykluszeit1, Zykluszeit2A, Zykluszeit2B"(w605) -> ()
          n177 = Index Array(array=w610, index=1 ("Index")) -> (element=w608:i32)
          n178 = Add(x=w608, y=w607) -> (x+y=w606:i32)
          "Zyklnum1ges" <- w606
        }
        n179 = local read "ZwangsFPGABoolesch?"() -> (w513:bool[])
        n180 = Build Cluster Array(w507, w502, w501, w500) -> (w532:cluster{"HorstSPMod2B":dbl[][]}[])
        n181 = Build Cluster Array(w552, w551, w550, w549) -> (w534:cluster{"DIOsSPMod2B":bool[][]}[])
        n182 = Build Cluster Array(w548, w547, w546, w545) -> (w535:cluster{"ZeitpktDIOsMod2B":dbl[]}[])
        n183 = Build Cluster Array(w556, w555, w554, w553) -> (w533:cluster{"Mod2BHorstZeitpkt":dbl[]}[])
        n184 = Index Array(array=w507, index (row)=0 ("Index (Zeile)")) -> (element=w499:dbl[])  [unwired: 1 in]
        n185 = Index Array(array=w502, index (row)=0 ("Index (Zeile)")) -> (element=w498:dbl[])  [unwired: 1 in]
        n186 = Index Array(array=w501, index (row)=0 ("Index (Zeile)")) -> (element=w497:dbl[])  [unwired: 1 in]
        n187 = Index Array(array=w500, index (row)=0 ("Index (Zeile)")) -> (element=w496:dbl[])  [unwired: 1 in]
        n188 = local read "ZwangsHorst?"() -> (w515:cluster{bool[]}[])
        n189 = local read "ZwangsDIO?"() -> (w517:cluster{bool[]}[])
        n190 = Bundle(w535, w534, w533, w532, "LHHeizen?"=w531, "ZPktFPGABoolesch"=w530, "FPGABoolesch"=w529, "ZeitpktFPGAPID"=w528, "FPGAPID"=w527, "ZeitpktFPGAFixp"=w526, "FPGAFixp"=w525, "ZeitpktMach1"=w524, "TempMach1"=w523, "ZeitpktMach2"=w522, "TempMach2"=w521) -> (w520:T15)  [unwired: 1 in]
        n191 = Bundle("Zyklusnummern 0, 1, 2A, 2B"=w519, "ZeilennummernDIOs"=w518, "ZwangsDIO?"=w517, "ZeilennummernHorst"=w516, "ZwangsHorst?"=w515, "ZeileFPGABoolesch"=w514, "ZwangsFPGABoolesch?"=w513, "ZeileFPGAPID"=w512, "ZeileFPGAFixp"=w511, "ZeileMach1"=w510, "ZeileMach2"=w509) -> (w508:T16)  [unwired: 1 in]
        n192 = Build Array (concatenate)(w499, w498, w497, w496) -> (w495:dbl[])
        n193 = while "ZyklusSteuerung" {
          tunnel: w564 -> [w594]
          tunnel: w563 -> [w595]
          shift-right: [w586] -> _
          shift-left: w495 -> [w585]
          shift-right: [w582] -> _
          shift-left: w508 -> [w581]
          tunnel: w520 -> [w580]
          stop <- w596 stop-if-true
          n194 = call "Warten13"("Count(mSec)"=u32 100) -> ()  [unwired: 1 out]
          n195 = local read "Methodenwechsel?"() -> (w600:bool)
          n196 = local read "veränderte Methode benutzen"() -> (w597:bool)
          n197 = local read "Zyklusnummern 0, 1, 2A, 2B"() -> (w584:i32[])
          n198 = global read "gvbooleschRT.vi" "global stop RT"() -> (w601:bool)
          n199 = local read "Zykluszeiten 0, 1, 2A, 2B"() -> (w593:dbl[])
          n200 = local read "ZwangsFPGABoolesch?"() -> (w579:bool[])
          n201 = local read "ZwangsFPGABoolesch!"() -> (w588:bool[])
          n202 = local read "ZwangsLangsameH?"() -> (w590:bool[])
          n203 = local read "ZwangsLangsameH!"() -> (w589:bool[])
          n204 = local read "ZwangsHorst?"() -> (w583:cluster{bool[]}[])
          n205 = local read "ZwangsHorst!"() -> (w591:cluster{dbl[]}[])
          n206 = local read "ZwangsDIO?"() -> (w578:cluster{bool[]}[])
          n207 = local read "ZwangsDIO!"() -> (w592:cluster{bool[]}[])
          n208 = Or(x=w600, y=w601) -> (x .or. y?=w598:bool)
          n209 = Or(x=w598, y=w597) -> (x .or. y?=w596:bool)
          n210 = call "Zyklussteuerung.vi"("FPGA VI Reference In"=w595, "DIOsNummern"=w594, "Zyklusnummern 0, 1, 2A, 2B"=w584, "Zykluszeiten 0, 1, 2A, 2B"=w593, "Zeitpkte/SPs"=w580, "HorstSP"=w585, "ZwangsDIO?"=w578, "ZwangsLangsameH?"=w590, "ZwangsDIO!"=w592, "ZwangsLangsameH!"=w589, "ZwangsHorst?"=w583, "ZwangsFPGABoolesch?"=w579, "ZwangsHorst!"=w591, "ZwangsFPGABoolesch!"=w588, "Schieberegister"=w581) -> ("HorstSP"=w586:dbl[], "Heizen?LH"=w587:bool[], "Schieberegister"=w582:T17)  [unwired: 2 in]
          "HorstSP" <- w586
          n211 = local write "Heizen?LH"(w587) -> ()
        }
        n212 = global read "gvbooleschRT.vi" "global stop RT"() -> (w574:bool)
      }
      n213 = while {
        tunnel: w203 -> [w409]
        stop <- w413 stop-if-true
        n214 = local read "Big Ben, Methodenzeit, Zykluszeit0, Zykluszeit1, Zykluszeit2A, Zykluszeit2B"() -> (w403:dbl[])
        n215 = call "Warten20"("Count(mSec)"=u32 1000) -> ()  [unwired: 1 out]
        n216 = local read "Zyklusnummern 0, 1, 2A, 2B"() -> (w405:i32[])
        n217 = local read "Mod1Mod2Mod3/AITrapsMachs1Hz"() -> (w402:dbl[])
        n218 = local read "Zyklnum1ges"() -> (w407:i32)
        n219 = local read "Probenvol.1"() -> (w400:dbl)
        n220 = local read "Probenvol.2"() -> (w399:dbl)
        n221 = local read "MWHorst"() -> (w401:dbl[])
        n222 = local read "aktuelle TDMS-Datei"() -> (w410:refnum<k34>)
        n223 = To Double Precision Float(number=w407) -> (double precision float=w406:dbl)
        n224 = To Double Precision Float(number=w405) -> (double precision float=w404:dbl[])
        n225 = global read "gvbooleschRT.vi" "global stop RT"() -> (w413:bool)
        n226 = Build Array (concatenate)(w406, w404, w403, w402, w401, w400, w399) -> (w408:dbl[])
        n227 = TDMS Write(0:w410, 1:enum16{"decimated", "interleaved"}."interleaved" ("Daten-Layout (0:dezimiert)"), 7:w409, 9:w408) -> ()  [unwired: 2 in, 4 out]
      }
      n228 = while {
        tunnel: path "c:/fromcriocmd.txt" ("Dateipfad (Dialog verwenden)") -> [w449]
        tunnel: w208 -> [w450]
        stop <- w451 stop-if-true
        n229 = local read "Dateien fürs MS schicken?"() -> (w448:bool)
        n230 = global read "gvbooleschRT.vi" "global stop RT"() -> (w447:bool)
        n231 = local read "Zyklnum1ges"() -> (w437:i32)
        n232 = local read "Datum/Zeit"() -> (w438:string)
        n233 = Not(x=w447) -> (.not. x?=w446:bool)
        n234 = Boolean To (0,1)(Boolean=w446) -> (0, 1=w444:i16)
        n235 = call "MSDateienSchicken.vi"("Dateipfad:fromcriocmd"=w449, "Speicherlänge"="Speicherlänge", "wie wird gespeichert?"="wie wird gespeichert?", "Dateipfad:fromcriordy"=w450, "Datum/Zeit"=w438, "Dateien fürs MS schicken?"=w448, "Zyklnum1ges"=w437, "Info"="Info") -> ()  [unwired: 8 in]
        n236 = To Unsigned Long Integer(number=w444) -> (unsigned 32bit integer=w443:u32)
        n237 = global read "gvbooleschRT.vi" "global stop RT"() -> (w451:bool)
        n238 = Multiply(x=u32 10000 ("Zu wartende ms"), y=w443) -> (x*y=w442:u32)
        n239 = call "Warten11"("Count(mSec)"=w442) -> ()  [unwired: 1 out]
      }
      n240 = Index Array(array=w169, index #1=0 ("Index"), index #2=1 ("Index"), index #3=2 ("Index"), index #4=3 ("Index")) -> (element #1=w162:i32, element #2=w161:i32, element #3=w164:i32, element #4=w163:i32)
      n241 = Add(x=w164, y=w163) -> (x+y=w160:i32)
      n242 = Build Array(w162, w161, w160) -> (w159:i32[])
      n243 = for {
        N: 1 -> [_]
        tunnel: w149 -> [w376]
        tunnel: [w376] -> w153
        n244 = call "Warten8"("Count(mSec)"=u32 100) -> ()  [unwired: 1 out]
      }
      n245 = Index Array(array=w159, index #1=0 ("Index"), index #2=1 ("Index")) -> (element #1=w182:i32, element #2=w180:i32)
      n246 = Split 1D Array(array=w156, index=w182) -> (first subarray=w189:string[], second subarray=w191:string[])
      n247 = Split 1D Array(array=w158, index=w182) -> (first subarray=w186:dbl[], second subarray=w190:dbl[])
      n248 = Split 1D Array(array=w157, index=w182) -> (first subarray=w179:string[], second subarray=w181:string[])
      n249 = Add Array Elements(numeric array=w159) -> (sum=w170:i32)
      n250 = Split 1D Array(array=w190, index=w180) -> (first subarray=w185:dbl[], second subarray=w184:dbl[])
      n251 = Split 1D Array(array=w191, index=w180) -> (first subarray=w188:string[], second subarray=w187:string[])
      n252 = Split 1D Array(array=w181, index=w180) -> (first subarray=w178:string[], second subarray=w177:string[])
      n253 = Bundle(w189, w188, w187, w186, w185, w184) -> (w183:T18)  [unwired: 1 in]
      n254 = Bundle(w179, w178, w177) -> (w176:cluster{string[], string[], string[]})  [unwired: 1 in]
      n255 = Bundle(w173, w173, w173) -> (w172:cluster{string[], string[], string[]})  [unwired: 1 in]
      n256 = Initialize Array(-1.0 ("Element"), w170) -> (w154:dbl[])
      n257 = Bundle(w175, w175, w175) -> (w174:cluster{i32, i32, i32})  [unwired: 1 in]
      n258 = while {
        shift-right: [w362] -> _
        shift-left: bool[] [TRUE, TRUE, TRUE] -> [w350]
        shift-right: [w340] -> _
        shift-left: w154 -> [w355]
        tunnel: w153 -> [w351]
        shift-right: [w360] -> _
        shift-left: string[] ["", "", ""] -> [w361]
        shift-right: [w341] -> _
        shift-left: w154 -> [w359]
        tunnel: w155 -> [w358]
        tunnel: w158 -> [w357]
        shift-right: [w343] -> _
        shift-left: w172 -> [w345]
        tunnel: w182 -> [w353]
        tunnel: w180 -> [w354]
        tunnel: w183 -> [w356]
        tunnel: w176 -> [w348]
        shift-right: [w347] -> _
        shift-left: w174 -> [w349]
        stop <- w342 stop-if-true
        n259 = local read "HorstSP"() -> (w340:dbl[])
        n260 = Not Equal?(x=w340, y=w355) -> (x != y?=w346:bool)
        n261 = call "NeueSP.vi"("Anzahl2"=w354, "Anzahl1"=w353, "AlteSP"=w355, 7:"NeueSP"=w340, "BefehleCluster"=w345, 10:"NeueSP"=w346, "ClusterFest"=w356) -> ("BefehleCluster"=w344:T19)  [unwired: 4 in]
        n262 = call "Senden.vi"("FPGA VI Reference In"=w351, "BefehlsCluster"=w344, "Senden?"=w350, "Abfragenr.Cluster"=w349, "AbfragenCluster"=w348) -> ("Senden?"=w352:bool[], "Abfragenr.Cluster"=w347:cluster{i32, i32, i32}, "BefehlsCluster"=w343:T19)  [unwired: 1 in]
        n263 = global read "gvbooleschRT.vi" "global stop RT"() -> (w342:bool)
        n264 = call "SeriellRead.vi"("SkalierungsfaktorHorst"=w357, "VorwortHorst"=w358, 8:w359, "Zwischenspeicher"=w361, "Senden?"=w352, "FPGA VI Reference In"=w351) -> ("Senden?"=w362:bool[], "Zwischenspeicher"=w360:string[], 3:w341)  [unwired: 3 in]
        "MWHorst" <- w341
      }
      n265 = while {
        shift-right: [w379] -> _
        shift-left: w144 -> [w396]
        shift-right: [w383] -> _
        shift-left: w143 -> [w395]
        shift-right: [w382] -> _
        shift-left: w144 -> [w394]
        shift-right: [w378] -> _
        shift-left: w144 -> [w393]
        shift-right: [w381] -> _
        shift-left: w143 -> [w392]
        shift-right: [w380] -> _
        shift-left: w144 -> [w391]
        stop <- w398 stop-if-true
        n266 = local read "Zykluszeiten 0, 1, 2A, 2B"() -> (w386:dbl[])
        n267 = call "Warten22"("Count(mSec)"=u32 100) -> ()  [unwired: 1 out]
        n268 = local read "MWHorst"() -> (w385:dbl[])
        n269 = call "Integrieren.vi"(0:w396, "Integrieren1"=w395, "Integral1"=w394, 3:w393, "Integrieren2"=w392, "Integral2"=w391, "Int.Start1"="Int.Start1", 7:w386, "Int.Stop1"="Int.Stop1", 9:w385, "Int.Start2"="Int.Start2", "HorstProbenflußNr."="HorstProbenflußNr.", "Int.Stop2"="Int.Stop2") -> (14:w379, "Integrieren1"=w383:bool, "Integral1"=w382:dbl, 17:w378, "Integrieren2"=w381:bool, "Integral2"=w380:dbl)  [unwired: 1 in]
        "Probenvol.1" <- w379
        "Probenvol.2" <- w378
        n270 = global read "gvbooleschRT.vi" "global stop RT"() -> (w398:bool)
      }
      n271 = while {
        shift-right: [w677] -> w218
        shift-left: w221 -> [w678]
        shift-right: [w675] -> w217
        shift-left: w220 -> [w676]
        shift-right: [w672] -> _
        shift-left: 0 ("Zyklusnummer1") -> [w679]
        tunnel: w207 -> [w670]
        tunnel: w206 -> [w671]
        stop <- w681 stop-if-true
        n272 = local read "Zyklnum1ges"() -> (w672:i32)
        n273 = call "Warten2"("Count(mSec)"=u32 500) -> ()  [unwired: 1 out]
        n274 = local read "Methodennummer"() -> (w673:i32)
        n275 = Greater?(x=w672, y=w679) -> (0:w674:bool)
        n276 = call "AktuelleTDMS.vi"("AktuelleTDMS"=w678, "Dateiordner"=w671, "NächsteTDMS"=w676, "NeuerZyklus?"=w674, "Methodennummer"=w673, "Zyklnumges"=w672, "Dateiname"=w670) -> ("AktuelleTDMS"=w677:refnum<k34>, "NächsteTDMS"=w675:refnum<k34>)  [unwired: 5 in, 2 out]
        "aktuelle TDMS-Datei" <- w677
        n277 = global read "gvbooleschRT.vi" "global stop RT"() -> (w681:bool)
      }
    }
    frame #2 {
      n278 = TDMS Close(11:w693) -> ()  [unwired: 1 in, 2 out]
      n279 = TDMS Close(11:w692) -> ()  [unwired: 1 in, 2 out]
      n280 = local read "Ausgang"() -> (w688:T2)
      n281 = xnode "Read/Write Control"("FPGA VI Reference In"=w691, "global stop"=TRUE) -> ("FPGA VI Reference Out"=w690:refnum<k20>)  [unwired: 1 in, 1 out]
      n282 = Build Array(w688) -> (w687:T1)
      n283 = local write "Eingang"(w687) -> ()
      n284 = xnode "Close FPGA VI Reference"("FPGA VI Reference In"=w690) -> ()  [unwired: 1 in, 1 out]
    }
  }
